vi "Dashboard Main.vi"() -> ()   [LabVIEW 2016]
uses:
  <vilib>/vision/Image Controls.llb/IMAQ Image.ctl
  Dashboard Tabs.ctl
  <vilib>/Utility/miscctls.llb/LVRowAndColumnTypeDef.ctl
  <vilib>/event_ctls.llb/eventvkey.ctl
  <vilib>/Rock Robotics/WPI/DriverStation/WPI_DriverStationRobotMode2.ctl
  <vilib>/Rock Robotics/Network Tables/NT Read Numeric Array.vi
  <vilib>/Rock Robotics/Network Tables/NT Read Boolean.vi
  <vilib>/Rock Robotics/Network Tables/NT Write Boolean.vi
  <vilib>/Rock Robotics/WPI/Dashboard/WPI_DashboardLogging Global.vi
  <vilib>/ptbypt/NI_PtbyPt.lvlib
  <vilib>/vision/NI_Vision_Development_Module.lvlib
panel:
  in  "output cluster":T2
  in  "Size Limit %":dbl=0.04
  in  "LED Color":T3={"Hue"={30.0, 150.0}, "Sat"={67.0, 194.28571428571428}, "Val"={49.0, 194.0}} {"Hue" scale=0.0..255.0 scale format="%#_3g"}
  in  "Camera 0 Brightness":dbl=5.0
  out "Camera Image 3":T1(plugin-control)
  out "Camera Image 2":T1(plugin-control)
  in  "Camera Settings Right":T4={"Frame Rate"=15, "Compression"=30, "Size"=2, "DB Camera Config"=FALSE} {"Frame Rate" scale=1.0..30.0; "Compression" scale=100.0..-1.0; "Size" items=["640x480", "320x240", "160x120"]}
  in  "Camera Name Right":string(combo)="Camera1"
  out "Camera Info":cluster{"Mbps LED":bool, "Mbps":dbl, "fps":dbl}={"Mbps LED"=FALSE, "Mbps"=0.1809963067335802, "fps"=11.600928074245939} {"fps" format="%#.1g"; "Mbps" format="%#.1g"}
  in  "Camera Settings":T4={"Frame Rate"=15, "Compression"=30, "Size"=2, "DB Camera Config"=FALSE} {"Frame Rate" scale=1.0..30.0; "Compression" scale=100.0..-1.0; "Size" items=["640x480", "320x240", "160x120"]}
  in  "TCP":refnum<k5>
  in  "Rec Mode":enum32{"Stop", "Record", "Playback"}(radio)
  out "Robot IP":string="10.10.38.2"
  out "Image Message":string="Timeout in Camera Communications"
  in  "Dashboard Tab":T5(tab)=enum."Cooler Stuff"
  in  "Select Auto":string(combo)="Select Autonomous ..."
  out "NT Connection":bool=TRUE
  out "MotorChart R":cluster{"Numeric":dbl, "Numeric":dbl}(graph)
  out "MotorChart L":cluster{"Numeric":dbl, "Numeric":dbl}(graph)
  out "MotorSliders R":cluster{"MotorSlide1":dbl, "MotorSlide2":dbl} {"MotorSlide2" scale=-1.0..1.0 scale format="%#_2e"; "MotorSlide1" scale=-1.0..1.0 scale format="%#_2e"}
  out "MotorSliders L":cluster{"MotorSlide1":dbl, "MotorSlide2":dbl} {"MotorSlide2" scale=-1.0..1.0 scale format="%#_2e"; "MotorSlide1" scale=-1.0..1.0 scale format="%#_2e"}
  out "Gyro":dbl(knob)=346.0 scale=0.0..360.0
  out "JS1 Z":dbl(slide) scale=-1.0..1.0 scale format="%#_2e"
  out "JS1 Graph":cluster{"X":dbl, "Y":dbl}[](graph)
  out "JS1 Buttons":T6
  out "JS2 Z":dbl(slide) scale=-1.0..1.0 scale format="%#_2e"
  out "JS2 Graph":cluster{"X":dbl, "Y":dbl}[](graph)=[{"X"=0.0, "Y"=-0.007874015748031496}]
  out "JS2 Buttons":T6
  out "Mode":T7(ring)
  in  "Recalibrate Gyro":bool
  in  "DB/String 9":string
  in  "DB/String 8":string
  in  "DB/String 7":string
  in  "DB/String 6":string
  in  "DB/String 5":string
  in  "DB/String 4":string
  in  "DB/String 3":string
  in  "DB/String 2":string
  in  "DB/String 1":string
  in  "DB/String 0":string
  in  "DB/Slider 0":dbl(slide) scale=0.0..5.0
  in  "DB/Slider 1":dbl(slide) scale=0.0..5.0
  in  "DB/Slider 2":dbl(slide) scale=0.0..5.0
  in  "DB/Slider 3":dbl(slide) scale=0.0..5.0
  out "DB/LED 3":bool
  out "DB/LED 2":bool
  out "DB/LED 1":bool
  out "DB/LED 0":bool
  in  "DB/Button 3":bool
  in  "DB/Button 2":bool
  in  "DB/Button 1":bool
  in  "DB/Button 0":bool caption="New Name"
  out "Results":T8 {"Score" format="%#_3g"; "Pixels"."Rectangle"."Numeric 5" format="%#_3g"; "Pixels"."Rectangle"."Numeric 3" format="%#_3g"; "Pixels"."Rectangle"."Numeric 2" format="%#_3g"; "Pixels"."Rectangle"."Numeric" format="%#_3g"; "Normalized"."Rectangle"."Numeric 5" format="%#_2g"; "Normalized"."Rectangle"."Numeric 3" format="%#_2g"; "Normalized"."Rectangle"."Numeric 2" format="%#_2g"; "Normalized"."Rectangle"."Numeric" format="%#_2g"; "Normalized"."Center"."?" format="%#_3g"; "Normalized"."Center"."?" format="%#_3g"; "Distance (ft)" format="%#_3g"}
  in  "Test Slider":dbl(slide) scale=0.0..100.0 scale format="%#_3g"
  in  "On/Off":bool caption="Solenoid"
  in  "Test Name":u16(ring) items=["Select the test to run..."]
  in  "Test Tree":string(tree)
  in  "Motor":cluster{"Value":dbl, "Enable":bool} {"Value" scale=-1.0..1.0 scale format="%#_3g"}
  out "Progress":T9 {"Test Progress" scale=0.0..100.0}
  in  "Rev/Fwd":cluster{"Forward":bool, "Reverse":bool}
  in  "Test Ring":u16(ring) items=["Monochrome", "Color"]
  out "Cmd Status":string
  in  "Execute Command":bool
  in  "Command Params":string[][](table)
  in  "Command Selection":i32(listbox)
  in  "CheckList":i32(listbox)
  out "Tree":string(tree)
  out "Ultrasonic (in.)":dbl
  in  "PID Shooter Baseline":dbl=0.62
  in  "Shooter Baseline":dbl=0.62
  in  "PID Shooter RPS":dbl=40.0
  out "Left Shooter Speed":dbl
  out "Gyro Value":dbl(knob)=346.0 scale=0.0..360.0
  out "Gear Door":bool
  out "PTO":bool
  out "Shooting Motor":bool
  out "Right Drive Speed":dbl
  out "Left Drive Speed":dbl
  out "Drive Mode":string="Dual Stick Arcade"
  out "Right Shooter Speed":dbl
  in  "Gyro Reset":bool
  out "Vision Particles":dbl
  out "Added Power":dbl=0.0007874015748031496 format="%#.2f"
  out "Shooter Mode":string="Raw Control"
  out "Right Motor:":dbl
  out "Conveyor":bool
  out "Shooting":bool
  out "Should this tab be open":bool
  out "Left Motor:":dbl
  out "Gyro Angle":dbl=346.0
  in  "Auton Select":T10(ring)
  out "Vision Particles: Auton":dbl
  out "Camera Image":T1(plugin-control)
  out "Background":bool
  in  "Camera Name":string(combo)="Camera0"
  # "HW"
  # "HW"
  # "Joysticks"
  # "Drive Motors"
  # "Front"
  # "Right"
  # "Left"
  # "Back"
  # "This tab is a great place for autonomous settings and robot-specific values.\nPlace controls and indicators inside this tab and match name to\nDashboard Variables on robot. You can also delete this comment."
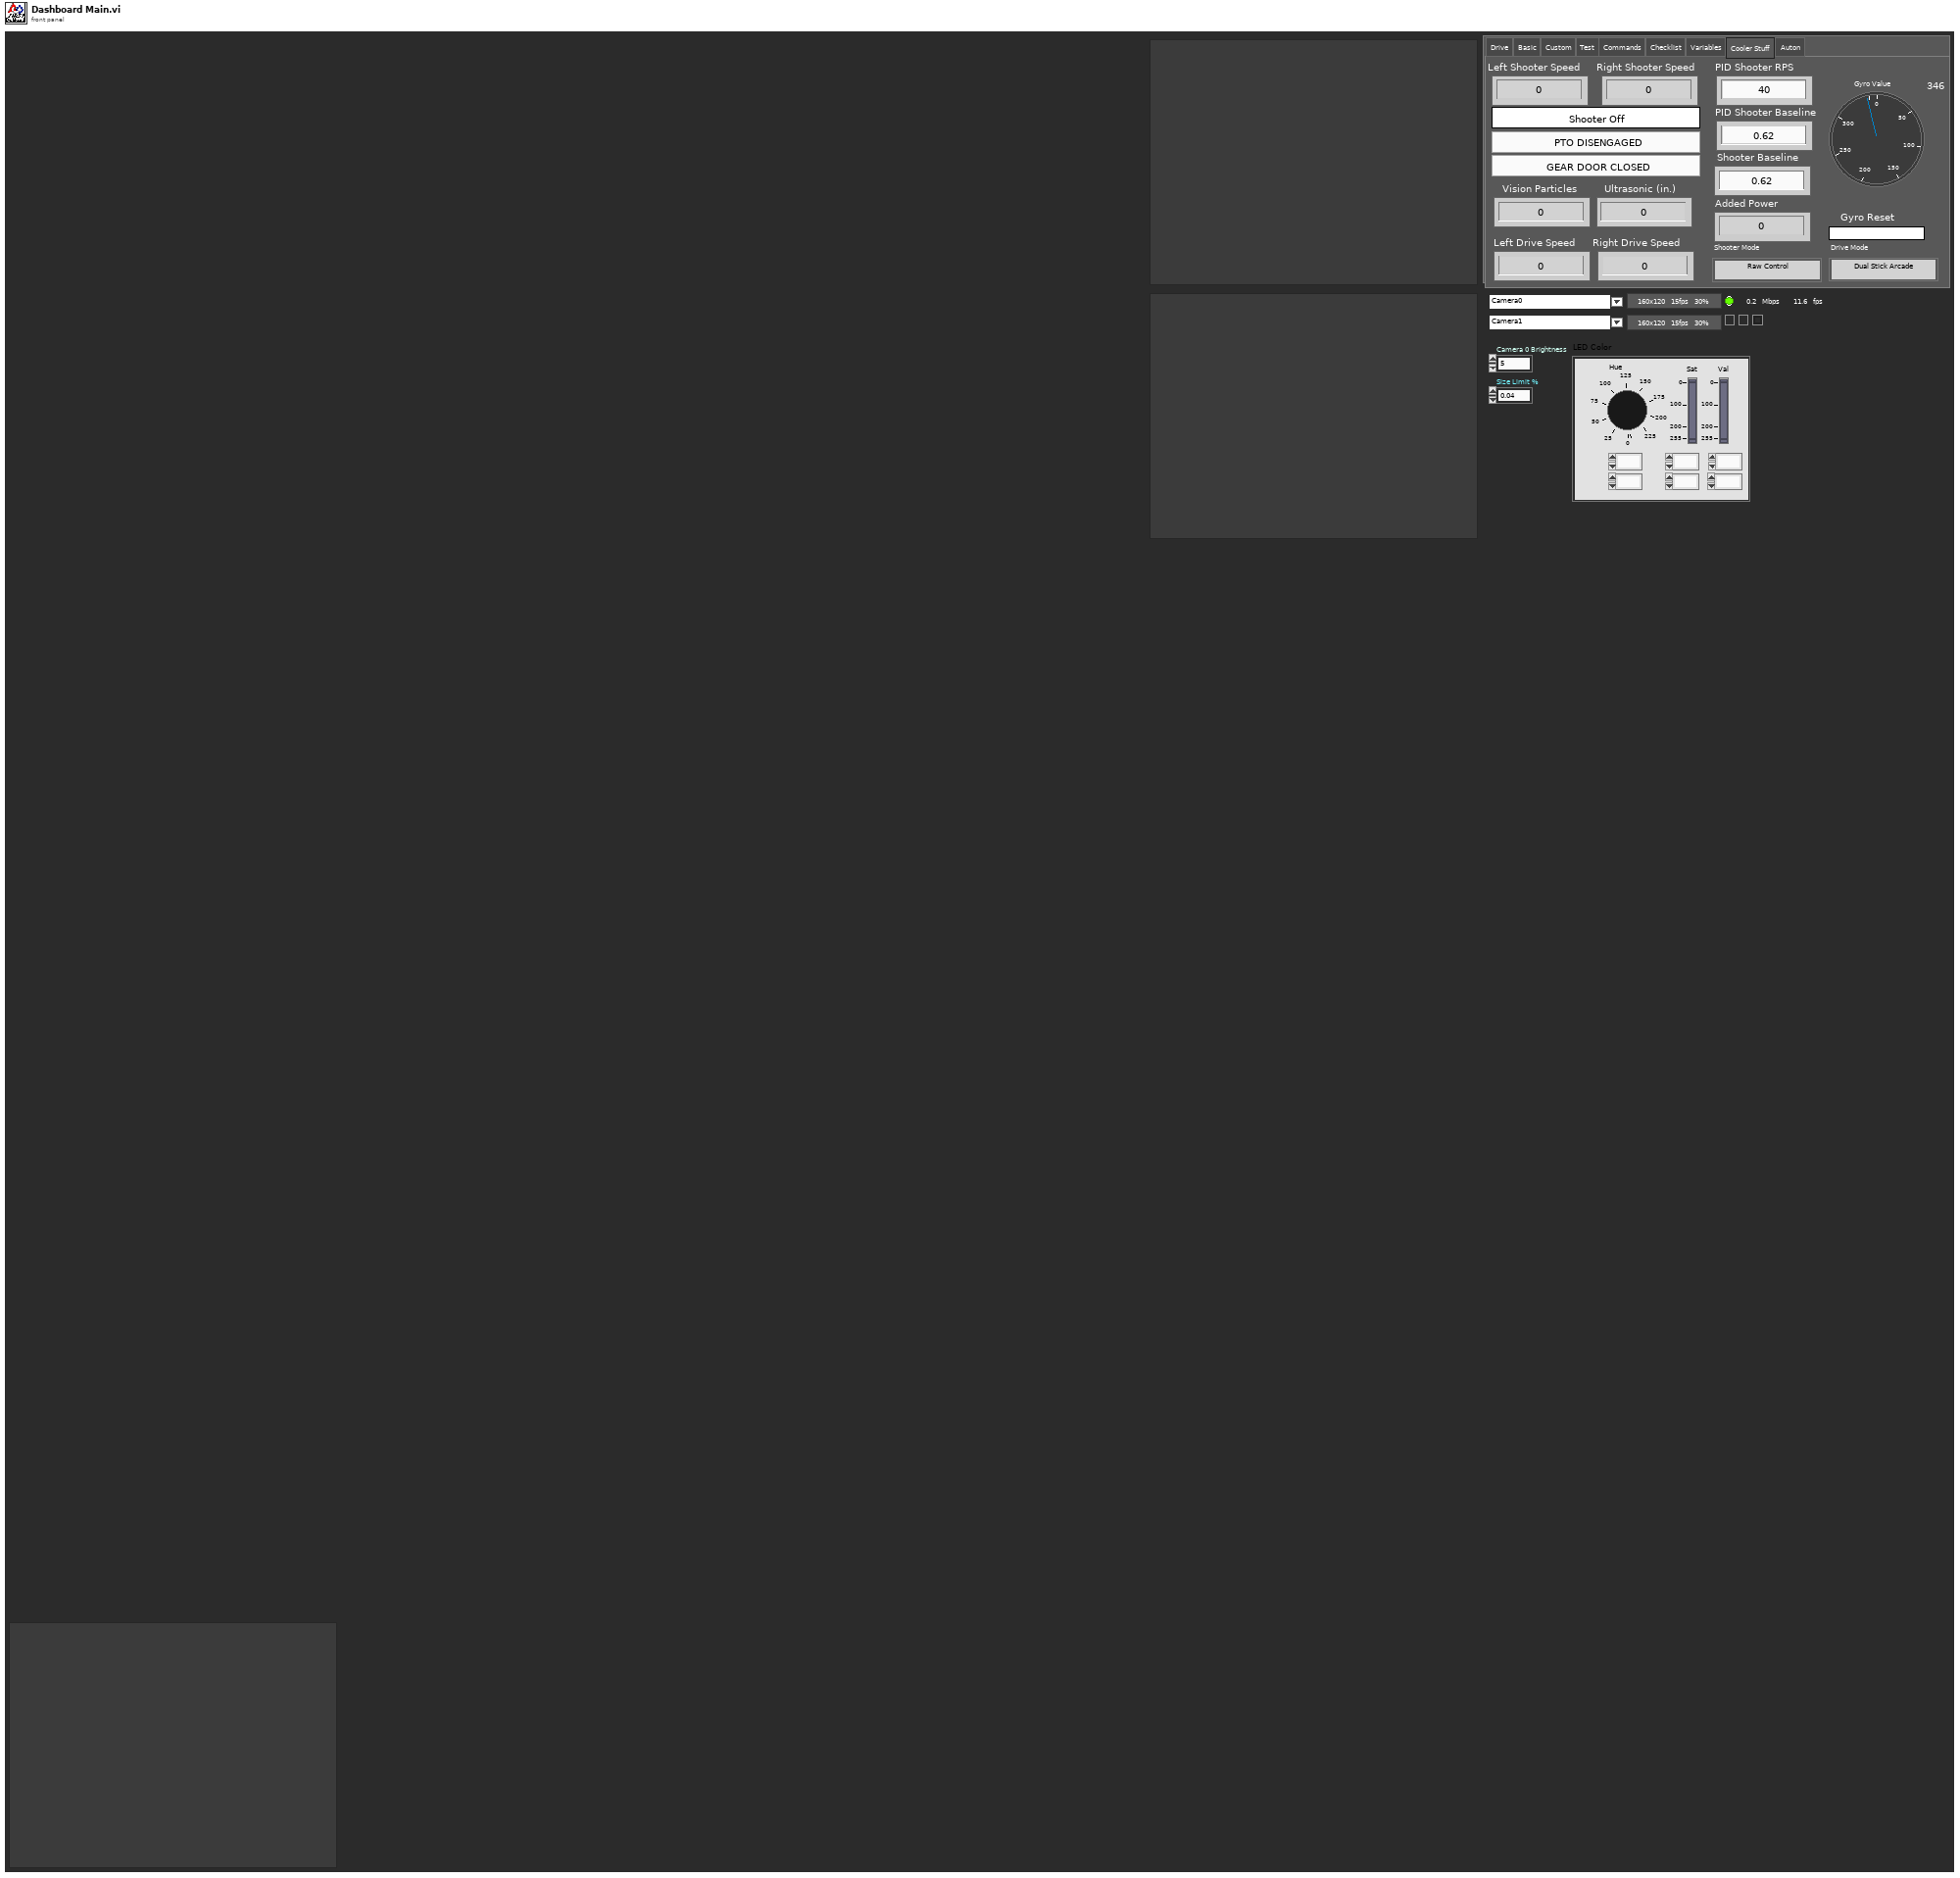
[diagram p1: front panel]
types:
  T1 = typedef "IMAQ Image.ctl" = refnum<image>
  T2 = cluster{"Image out":T1, "Results":cluster{"Distance (ft)":dbl, "Score":dbl, "Normalized":cluster{"Center":cluster{dbl, dbl}, "Rectangle":cluster{"Numeric":dbl, "Numeric 2":dbl, "Numeric 3":dbl, "Numeric 5":dbl}}, "Pixels":cluster{"Center":cluster{dbl, dbl}, "Rectangle":cluster{"Numeric":dbl, "Numeric 2":dbl, "Numeric 3":dbl, "Numeric 5":dbl}}}, "Edges":cluster{"X":sgl, "Y":sgl}[]}
  T3 = cluster{"Hue":cluster{dbl, dbl}, "Sat":cluster{dbl, dbl}, "Val":cluster{dbl, dbl}}
  T4 = cluster{"Frame Rate":i32, "Compression":i32, "Size":u16, "DB Camera Config":bool}
  T5 = enum32{"Drive", "Basic", "Custom", "Test", "Commands", "Checklist", "Variables", "Cooler Stuff", "Auton "}
  T6 = cluster{bool, bool, bool, bool, bool, bool, bool, bool, bool, bool, bool, bool}
  T7 = enum8{"Tele-Op Disabled", "Tele-Op Enabled", "Auto Disabled", "Auto Enabled", "Test Disabled", "Test Enabled", "Disconnected", "No Code", "E-Stop"}
  T8 = cluster{"Distance (ft)":dbl, "Score":dbl, "Normalized":cluster{"Center":cluster{dbl, dbl}, "Rectangle":cluster{"Numeric":dbl, "Numeric 2":dbl, "Numeric 3":dbl, "Numeric 5":dbl}}, "Pixels":cluster{"Center":cluster{dbl, dbl}, "Rectangle":cluster{"Numeric":dbl, "Numeric 2":dbl, "Numeric 3":dbl, "Numeric 5":dbl}}}
  T9 = cluster{"Test Progress":u8, "Test Progress Text":string}
  T10 = enum16{"Nothing", "Boiler Gear Auton", "Far Gear Auton", "Center Gear Auton", "Center Gear No Vision", "Center Gear Baseline Left", "Boiler Shoot", "Center Shoot", "Boiler Gear Shoot", "Center Gear Shoot", "Boiler Bucket Shoot", "Far Gear Bucket Cross", "Drive Straight"}
  T11 = typedef "Dashboard Tabs.ctl" = enum32{"Drive", "Basic", "Custom", "Test", "Commands", "Checklist", "Variables", "Cooler Stuff", "Auton "}
  T12 = typedef "Image Type" = u32
  T13 = cluster{"IDs":cluster{"RPC field ID":u16, "Unique ID":u16}, "String":string}
  T14 = enum32{"Drive", "Basic", "Custom", "Test", "Checklist", "Variables"}
  T15 = typedef "WPI_DriverStationRobotMode2.ctl" = enum16{"Autonomous Disabled", "Autonomous Enabled", "Teleop Disabled", "Teleop Enabled", "Disconnected", "Finish", "Test Disabled", "Test Enabled", "Emergency Stopped"}
  T16 = cluster{"Error Strings":string, "Disable Counts":cluster{u16, u16}, "Rail Faults":cluster{u16, u16, u16}, "Robot IP":string, "DB Mode":u8, "Event Info":cluster{"Name":string, "Type":u8, "Number":u16, "Replay":u8}}
  T17 = cluster{"Storage":cluster{"Disk Free":u64, "RAM Block":u32, "RAM free":u32}, "CPU Utilization":cluster{"CPU % ISR":sgl, "CPU % Time Crit":sgl, "CPU % Timed Str":sgl, "CPU % High":sgl, "CPU % Above":sgl, "CPU % Normal":sgl, "CPU % Low":sgl}, "CAN":cluster{"% Bus Utilization":sgl, "Bus Off Cnt":u32, "TX_FIFO Full Cnt":u32, "Receive Error Cnt":u8, "Transmit Error Cnt":u8}, "HID":cluster{"HID Outputs":u32, "Rumble Low":u16, "Rumble High":u16}[]}
  T18 = cluster{"Status bits":cluster{"Test Mode":bool, "Autonomous":bool, "Enabled":bool, "Code Start":bool, "Brownout":bool, "Reserved 2":bool, "Reserved 3":bool, "E-Stop":bool}, "Code Trace":cluster{"Disabled":bool, "TeleOp":bool, "Auto":bool, "Test":bool}, "Controller Type":enum16{"unknown", "cRIO", "roboRio"}, "Code?":enum16{"unknown", "noCode", "code"}, "Battery V":dbl}
  T19 = cluster{"Control Bits":cluster{"TestMode":bool, "Autonomous":bool, "Enabled":bool, "FMS Present":bool, bool, bool, bool, "E-Stop":bool}, "Team Station ":u8, "Countdown":sgl, "Joystick Values":cluster{"Axes":dbl[], "Buttons":bool[], "POVs":i16[]}[]}
  T20 = cluster{"Axes":dbl[], "Buttons":bool[], "POVs":i16[]}[]
  T21 = cluster{"Axes":dbl[], "Buttons":bool[], "POVs":i16[]}
  T22 = cluster{"Buttons[0]":bool, "Buttons[1]":bool, "Buttons[2]":bool, "Buttons[3]":bool, "Buttons[4]":bool, "Buttons[5]":bool, "Buttons[6]":bool, "Buttons[7]":bool, "Buttons[8]":bool, "Buttons[9]":bool, "Buttons[10]":bool, "Buttons[11]":bool}
  T23 = cluster{"Camera Image":refnum<vi>, "Dashboard Tab":refnum<vi>, "Background":refnum<vi>, "Rec Mode":refnum<vi>, "Test Slider":refnum<vi>, "On/Off ":refnum<vi>, "Test Ring":refnum<vi>, "Rev/Fwd":refnum<vi>, "Test Name":refnum<vi>, "Motor":refnum<vi>, "Progress":refnum<vi>, "CheckList":refnum<vi>, "Tree":refnum<vi>, "Test Tree":refnum<vi>, "Command Params":refnum<vi>, "Command Selection":refnum<vi>, "Execute Command":refnum<vi>, "Cmd Status":refnum<vi>, "Camera Settings":refnum<vi>, "Camera Name":refnum<vi>, "Camera Info":refnum<vi>, "Camera Settings Right":refnum<vi>, "Camera Name Right":refnum<vi>, "Camera Image":refnum<vi>}
  T24 = cluster{"Operation":enum16{"Update", "Clear"}, "Color Box":u32}[]
  T25 = typedef "eventvkey.ctl" = enum16{"ASCII", "Enter", "Return", "Shift", "Ctrl", "Alt", "Cmd", "Opt", "Caps", "NumLock", "Clear", "Break", "Up", "Down", "Left", "Right", "Insert", "Delete", "Home", "End", "PageUp", "PageDown", "Escape", "Help", "Pause", "ScrollLock", "F1", "F2", "F3", "F4", "F5", "F6", "F7", "F8", "F9", "F10", "F11", "F12", "F13", "F14", "F15", "F16", "F17", "F18", "F19", "F20", "F21", "F22", "F23", "F24", "Play", "VolumeUp", "VolumeDown", "Mute", "Two Byte Char"}
  T26 = cluster{"Image Size":bool, "Image Type":bool, "Pixel Value":bool, "ROI Information":bool, "Zoom Factor":bool}
  T27 = cluster{"Operation":enum16{"Update", "Clear"}, "Color Box":u32}
  T28 = typedef "LVRowAndColumnTypeDef.ctl" = cluster{"Row":i32, "Column":i32}
  T29 = cluster{"Shift":bool, "Ctrl":bool, "Alt":bool, "Cmd":bool, "Opt":bool}
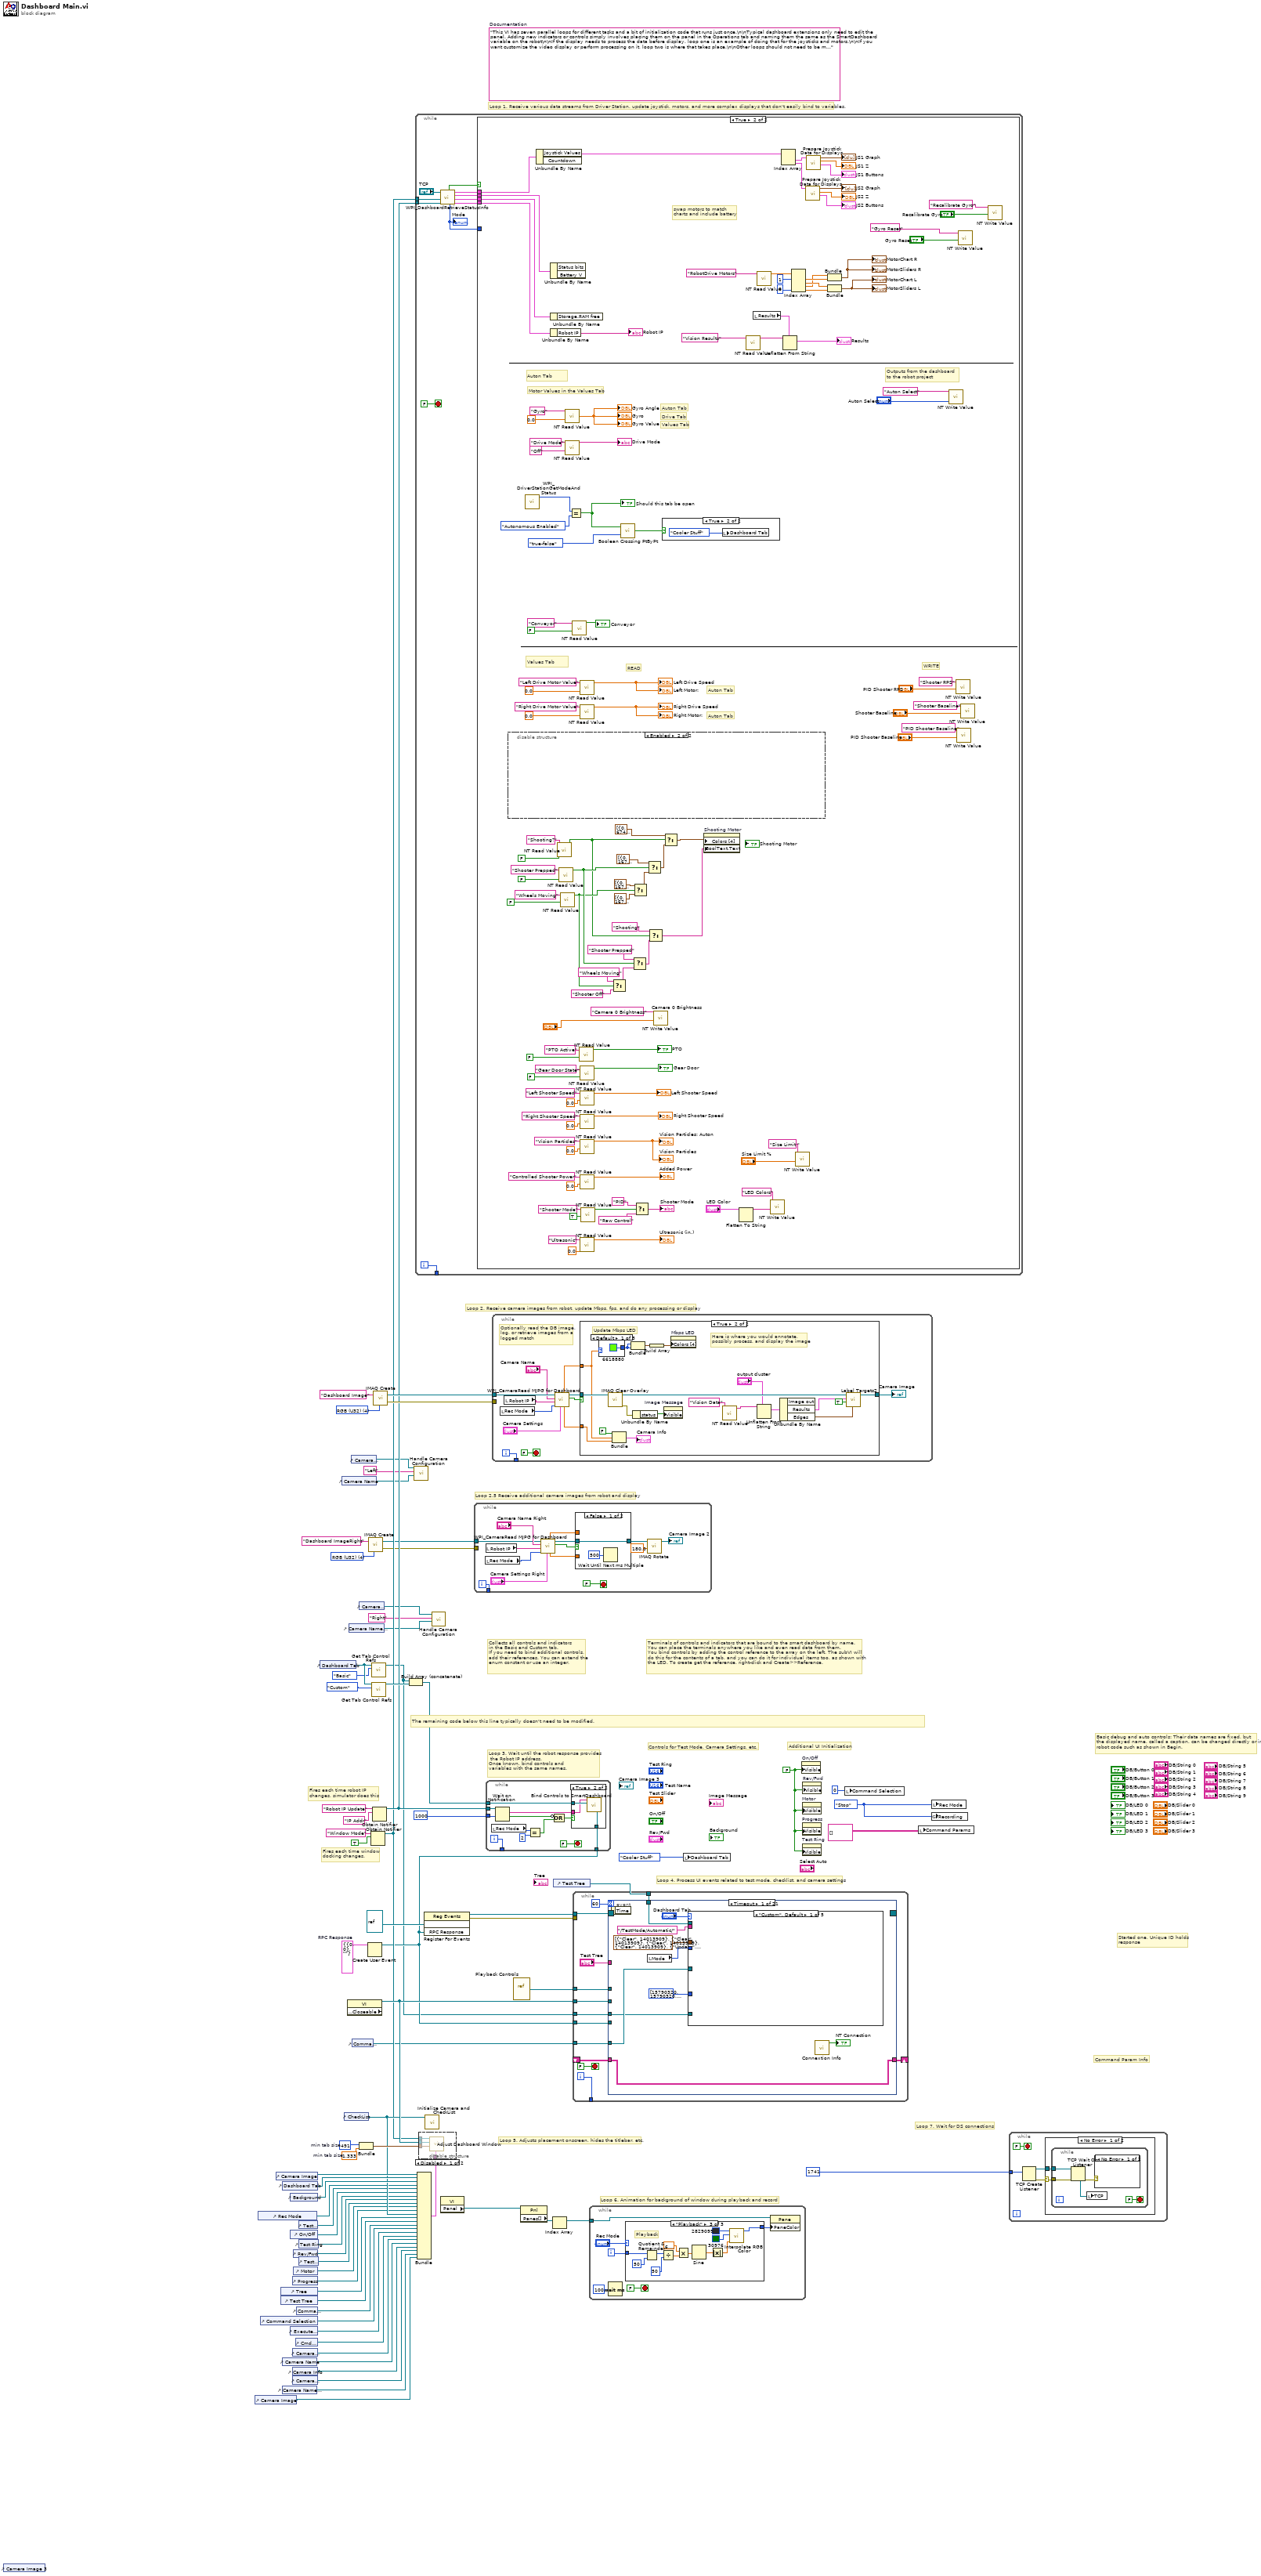
[diagram p0: block diagram]
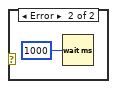
[diagram p4: hidden frame]
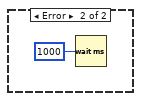
[diagram p5: hidden frame]
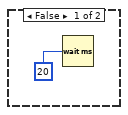
[diagram p6: hidden frame]
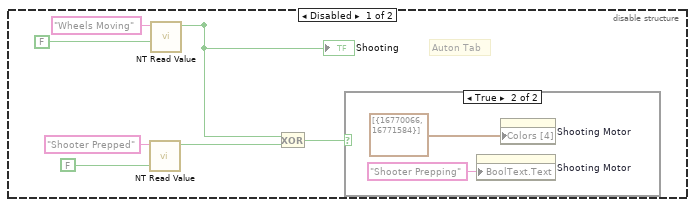
[diagram p7: hidden frame]
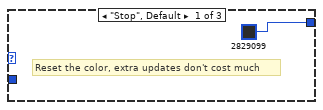
[diagram p10: hidden frame]
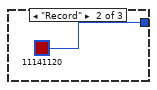
[diagram p11: hidden frame]
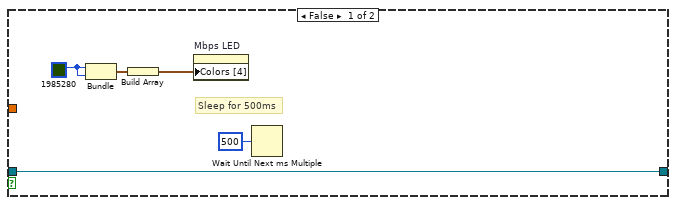
[diagram p13: hidden frame]
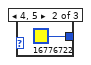
[diagram p14: hidden frame]
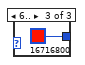
[diagram p15: hidden frame]
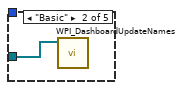
[diagram p16: hidden frame]
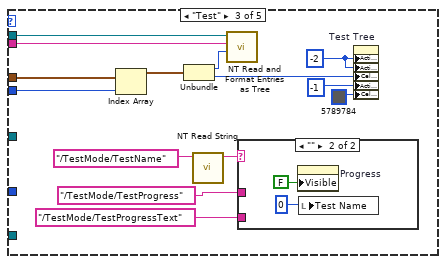
[diagram p17: hidden frame]
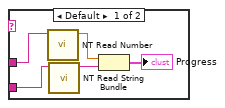
[diagram p18: hidden frame]
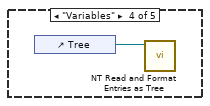
[diagram p19: hidden frame]
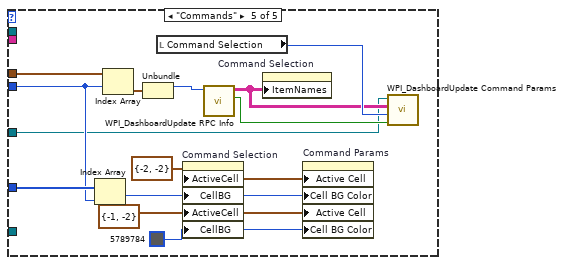
[diagram p20: hidden frame]
diagram:
  w11 = T12 4 items=["Grayscale (U8)", "Grayscale (I16)", "Grayscale (SGL)", "Complex (CSG)", "RGB (U32)", "HSL (U32)", "RGB (U64)"] ("Image Type")
  w25 = T13 {"IDs"={"RPC field ID"=0, "Unique ID"=0}, "String"=""}  # RPC Response
  w49 = 491  # min tab size
  w48 = 1.333  # min tab size
  w56 = enum32{"Stop", "Record", "Playback"}."Stop" ("Rec Mode")
  w31 = FALSE ("Visible")
  (unwired) "This VI has seven parallel loops for different tasks and a bit of initialization code that runs just once.\n\nTypical dashboard extensions only need to edit the panel. Adding new indicators or controls simply involves placing them on the panel in the Operations tab and naming them the same as the SmartDashboard variable on the robot\n\nIf the display needs to process the data before display, loop one is an example of doing that for the joysticks and motors.\n\nIf you want customize the video display or perform processing on it, loop two is where that takes place.\n\nOther loops should not need to be modified. They are pretty standard, and document the task they perform."  # Documentation
  w73 = T12 4 items=["Grayscale (U8)", "Grayscale (I16)", "Grayscale (SGL)", "Complex (CSG)", "RGB (U32)", "HSL (U32)", "RGB (U64)"] ("Image Type")
  # "Loop 2.5 Receive additional camera images from robot and display"
  # "Command Param Info"
  # "Started one, Unique ID holds\nresponse"
  # "Loop 7. Wait for DS connections"
  # "Basic debug and auto controls: Their data names are fixed, but\nthe displayed name, called a caption, can be changed directly or in\nrobot code such as shown in Begin."
  # "Controls for Test Mode, Camera Settings, etc."
  # "Additional UI Initialization"
  # "Loop 6. Animation for background of window during playback and record"
  # "Fires each time robot IP\nchanges, simulator does this"
  # "Fires each time window\ndocking changes."
  # "Collects all controls and indicators\nin the Basic and Custom tab.\nIf you need to bind additional controls,\nadd their references. You can extend the\nenum constant or use an integer."
  # "The remaining code below this line typically doesn't need to be modified."
  # "Loop 4. Process UI events related to test mode, checklist, and camera settings"
  # "Terminals of controls and indicators that are bound to the smart dashboard by name.\nYou can place the terminals anywhere you like and even read data from them.\nYou bind controls by adding the control reference to the array on the left. The subVI will\ndo this for the contents of a tab, and you can do it for individual items too, as shown with\nthe LED. To create get the reference, right-click and Create>>Reference."
  # "Loop 3. Wait until the robot response provides\n the Robot IP address.\nOnce known, bind controls and\nvariables with the same names."
  # "Loop 5. Adjusts placement onscreen, hides the titlebar, etc."
  # "Loop 1. Receive various data streams from Driver Station, update joystick, motors, and more complex displays that don't easily bind to variables."
  # "Loop 2. Receive camera images from robot, update Mbps, fps, and do any processing or display"
  n1 = control-ref of="Camera Image 3"() -> ()  [unwired: 1 out]
  n2 = control-ref of="Camera Image"() -> (w2:refnum<vi>)
  n3 = control-ref of="Rec Mode"() -> (w37:refnum<vi>)
  n4 = control-ref of="Command Selection"() -> (w24:refnum<vi>)
  n5 = control-ref of="Camera Image"() -> (w51:refnum<vi>)
  n6 = control-ref of="Tree"() -> (w41:refnum<vi>)
  n7 = control-ref of="Test Tree"() -> (w40:refnum<vi>)
  n8 = control-ref of="Dashboard Tab"() -> (w50:refnum<vi>)
  n9 = control-ref of="Camera Name"() -> (w15:refnum<vi>)
  n10 = control-ref of="Camera Name Right"() -> (w3:refnum<vi>)
  n11 = control-ref of="Execute Command"() -> (w26:refnum<vi>)
  n12 = control-ref of="Background"() -> (w46:refnum<vi>)
  n13 = control-ref of="On/Off"() -> (w35:refnum<vi>)
  n14 = control-ref of="Progress"() -> (w32:refnum<vi>)
  n15 = control-ref of="Camera Settings"() -> (w16:refnum<vi>)
  n16 = control-ref of="Camera Info"() -> (w14:refnum<vi>)
  n17 = control-ref of="Camera Settings Right"() -> (w4:refnum<vi>)
  n18 = control-ref of="Rev/Fwd"() -> (w33:refnum<vi>)
  n19 = control-ref of="Motor"() -> (w38:refnum<vi>)
  n20 = control-ref of="Cmd Status"() -> (w20:refnum<vi>)
  n21 = control-ref of="Command Params"() -> (w27:refnum<vi>)
  n22 = control-ref of="Test Slider"() -> (w36:refnum<vi>)
  n23 = control-ref of="Test Ring"() -> (w34:refnum<vi>)
  n24 = control-ref of="Test Name"() -> (w39:refnum<vi>)
  n25 = control-ref of="Dashboard Tab"() -> (w54:refnum<vi>)
  n26 = control-ref of="Camera Name"() -> (w17:refnum<vi>)
  n27 = control-ref of="CheckList"() -> (w42:refnum<vi>)
  n28 = property class="VI" props=["Front Panel.Closeable"]() -> (reference out=w55:refnum<vi>)  [unwired: 2 in, 2 out]
  n29 = control-ref of="Camera Name Right"() -> (w7:refnum<vi>)
  n30 = control-ref of="Camera Settings"() -> (w18:refnum<vi>)
  n31 = control-ref of="Command Params"() -> (w19:refnum<vi>)
  n32 = control-ref of="Camera Settings Right"() -> (w8:refnum<vi>)
  n33 = Bundle("min tab size"=w49, "min tab size"=w48) -> (w47:cluster{"min tab size":i32, "min tab size":dbl})  [unwired: 1 in]
  n34 = Create User Event(user event datatype=w25) -> (user event=w21:refnum<user-event>)  [unwired: 1 in, 1 out]
  n35 = call "IMAQ Create"("Image Name"="Dashboard ImageRight", "Image Type"=w11) -> ("New Image"=w10:T1, "error out"=w9:errorcluster)  [unwired: 2 in, 1 out]
  n36 = Obtain Notifier(name (unnamed)="Window Mode", notification data type=TRUE) -> (notifier out=w29:refnum<notifier>)  [unwired: 2 in, 2 out]
  n37 = call <vilib>:"Get Tab Control Refs.vi"("Page Index"=T14."Basic" ("Dashboard Tab"), "TabControl in"=w54) -> ("ControlsOnPage"=w13:refnum<vi>[])  [unwired: 9 in]
  n38 = call <vilib>:"Get Tab Control Refs.vi"("Page Index"=T14."Custom" ("Dashboard Tab"), "TabControl in"=w54) -> ("ControlsOnPage"=w53:refnum<vi>[])  [unwired: 9 in]
  n39 = Obtain Notifier(name (unnamed)="Robot IP Update", notification data type="IP Addr" ("name (unnamed)")) -> (notifier out=w30:refnum<notifier>)  [unwired: 2 in, 2 out]
  n40 = call "IMAQ Create"("Image Name"="Dashboard Image", "Image Type"=w73) -> ("New Image"=w71:T1, "error out"=w70:errorcluster)  [unwired: 2 in, 1 out]
  n41 = Build Array (concatenate)(w13, w53) -> (w52:refnum<vi>[])
  n42 = call "Handle Camera Configuration.vi"("CameraNameRef"=w17, "Camera File Name"="Left", "ClusterRef"=w18) -> ()  [unwired: 9 in]
  n43 = while {
    tunnel: [w83] -> _
    tunnel: w30 -> [w77]
    tunnel: w29 -> [w74]
    i -> [w83]
    stop <- FALSE stop-if-true
    n44 = call <vilib>:"WPI_DashboardRetrieveStatusInfo.vi"("Binding Refnum"=w77, "Window Mode Notifier"=w74, "TCP Cnx"="TCP") -> ("Power and Errors"=w78:T16, "Robot Metrics"=w81:T17, "Status Info"=w82:T18, "Control Info"=w79:T19, "Robot Mode"=w76:T7, "Process?"=w80:bool)  [unwired: 3 in]
    "Mode" <- w76
    n45 = case shown="True" w80 {
      tunnel: w82 -> [_ w202]
      tunnel: w81 -> [_ w201]
      tunnel: w79 -> [_ w200]
      tunnel: w78 -> [_ w199]
      tunnel: w76 -> [_ _]
      frame False {
        n46 = Wait (ms)(milliseconds to wait=u32 20) -> ()  [unwired: 1 out]
      }
      frame True {
        # "WRITE"
        # "READ"
        # "Outputs from the dashboard \nto the robot project"
        # "Motor Values in the Values Tab"
        # "Auton Tab"
        # "Auton Tab"
        # "Values Tab"
        # "Auton Tab"
        # "Drive Tab"
        # "Values Tab"
        # "Auton Tab"
        # "swap motors to match\ncharts and include battery"
        n47 = disable-structure shown="Enabled" {
          frame Disabled {
            # "Auton Tab"
            n48 = call-poly <vilib>:"NT Read Value.vi"("Default Value"=FALSE, "Name"="Shooter Prepped") -> ("Boolean"=w204:bool)  [unwired: 8 in, 1 out]
            n49 = call-poly <vilib>:"NT Read Value.vi"("Default Value"=FALSE, "Name"="Wheels Moving") -> ("Boolean"=w205:bool)  [unwired: 8 in, 1 out]
            "Shooting" <- w205
            n50 = Exclusive Or(1:w204, 2:w205) -> (0:w203:bool)
            n51 = case shown="True" w203 {
              frame False {
              }
              frame True {
                n52 = property on="Shooting Motor" class="Bool (strict)"("BoolText.Text"="Shooter Prepping" ("Boolean Text.Text")) -> ()  [unwired: 2 in, 2 out]
                n53 = property on="Shooting Motor" class="Bool (strict)"("Colors [4]"=cluster{u32, u32}[] [{16770066, 16771584}]) -> ()  [unwired: 2 in, 2 out]
              }
            }
          }
          frame Enabled {
          }
        }
        n54 = call <vilib>:"WPI_DriverStationGetModeAndStatus.vi"() -> ("Robot Mode"=w119:T15)  [unwired: 10 in, 1 out]
        n55 = Unbundle By Name(w200) -> ("Joystick Values"=w190:T20)  [unwired: 1 out]
        n56 = Unbundle By Name(w202) -> ()  [unwired: 2 out]
        n57 = Unbundle By Name(w201) -> ()  [unwired: 1 out]
        n58 = Unbundle By Name(w199) -> ("Robot IP"=→"Robot IP":string)
        n59 = call-poly <vilib>:"NT Read Value.vi"("Default Value"=FALSE, "Name"="Shooting?") -> ("Boolean"=w126:bool)  [unwired: 8 in, 1 out]
        n60 = call-poly <vilib>:"NT Read Value.vi"("Default Value"=FALSE, "Name"="Shooter Prepped") -> ("Boolean"=w128:bool)  [unwired: 8 in, 1 out]
        n61 = call-poly <vilib>:"NT Read Value.vi"("Default Value"=FALSE, "Name"="Wheels Moving") -> ("Boolean"=w127:bool)  [unwired: 8 in, 1 out]
        n62 = call-poly <vilib>:"NT Read Value.vi"("Default Value"=0.0, "Name"="Gyro") -> ("Numeric"=→"Gyro" →"Gyro Angle" →"Gyro Value":dbl)  [unwired: 8 in, 1 out]
        n63 = call-poly <vilib>:"NT Read Value.vi"("Default Value"="Off", "Name"="Drive Mode") -> ("String"=→"Drive Mode":string)  [unwired: 8 in, 1 out]
        n64 = Equal?(x=w119, y=WPI_DriverStationRobotMode2."Autonomous Enabled" ("Robot Mode")) -> (x = y?=w118:bool)
        "Should this tab be open" <- w118
        n65 = call-poly <vilib>:"NT Read Value.vi"("Default Value"=FALSE, "Name"="Conveyor") -> ("Boolean"=→"Conveyor":bool)  [unwired: 8 in, 1 out]
        n66 = call-poly <vilib>:"NT Read Value.vi"("Default Value"=FALSE, "Name"="PTO Active") -> ("Boolean"=→"PTO":bool)  [unwired: 8 in, 1 out]
        n67 = call-poly <vilib>:"NT Read Value.vi"("Default Value"=0.0, "Name"="Left Drive Motor Value") -> ("Numeric"=→"Left Motor:" →"Left Drive Speed":dbl)  [unwired: 8 in, 1 out]
        n68 = call-poly <vilib>:"NT Read Value.vi"("Default Value"=0.0, "Name"="Right Drive Motor Value") -> ("Numeric"=→"Right Drive Speed" →"Right Motor:":dbl)  [unwired: 8 in, 1 out]
        n69 = call-poly <vilib>:"NT Read Value.vi"("Default Value"=FALSE, "Name"="Gear Door State") -> ("Boolean"=→"Gear Door":bool)  [unwired: 8 in, 1 out]
        n70 = call-poly <vilib>:"NT Read Value.vi"("Default Value"=0.0, "Name"="Left Shooter Speed") -> ("Numeric"=→"Left Shooter Speed":dbl)  [unwired: 8 in, 1 out]
        n71 = call-poly <vilib>:"NT Read Value.vi"("Default Value"=0.0, "Name"="Right Shooter Speed") -> ("Numeric"=→"Right Shooter Speed":dbl)  [unwired: 8 in, 1 out]
        n72 = call-poly <vilib>:"NT Read Value.vi"("Default Value"=0.0, "Name"="Vision Particles") -> ("Numeric"=→"Vision Particles: Auton" →"Vision Particles":dbl)  [unwired: 8 in, 1 out]
        n73 = call-poly <vilib>:"NT Read Value.vi"("Default Value"=0.0, "Name"="Controlled Shooter Power") -> ("Numeric"=→"Added Power":dbl)  [unwired: 8 in, 1 out]
        n74 = call-poly <vilib>:"NT Read Value.vi"("Default Value"=0.0, "Name"="Ultrasonic") -> ("Numeric"=→"Ultrasonic (in.)":dbl)  [unwired: 8 in, 1 out]
        n75 = call-poly <vilib>:"NT Read Value.vi"("Default Value"=TRUE, "Name"="Shooter Mode") -> ("Boolean"=w99:bool)  [unwired: 8 in, 1 out]
        n76 = Select(t="Wheels Moving", s=w127, f="Shooter Off") -> (s? t:f=w130:string)
        n77 = call <vilib>:"Boolean Crossing PtByPt.vi"("direction"=enum16{"either", "false-true", "true-false"}."true-false", "input"=w118) -> ("crossing"=w167:bool)  [unwired: 1 in]
        n78 = Select(t="Shooter Prepped", s=w128, f=w130) -> (s? t:f=w129:string)
        n79 = Select(t=cluster{u32, u32}[] [{0, 16728642}] ("Colors [4]"), s=w127, f=cluster{u32, u32}[] [{0, 16777215}] ("Colors [4]")) -> (s? t:f=w137:cluster{u32, u32}[])
        n80 = Select(t="PID", s=w99, f="Raw Control") -> (s? t:f=→"Shooter Mode":string)
        n81 = Select(t=cluster{u32, u32}[] [{0, 16776722}] ("Colors [4]"), s=w128, f=w137) -> (s? t:f=w136:cluster{u32, u32}[])
        n82 = Select(t="Shooting", s=w126, f=w129) -> (s? t:f=w125:string)
        n83 = call-poly <vilib>:"NT Write Value.vi"("Numeric"="Camera 0 Brightness", "Name"="Camera 0 Brightness") -> ()  [unwired: 9 in, 1 out]
        n84 = case shown="True" w167 {
          frame False {
          }
          frame True {
            n85 = local write "Dashboard Tab"(Dashboard_Tabs."Cooler Stuff" ("Dashboard Tab")) -> ()
          }
        }
        n86 = Select(t=cluster{u32, u32}[] [{0, 6749952}] ("Colors [4]"), s=w126, f=w136) -> (s? t:f=w131:cluster{u32, u32}[])
        n87 = property on="Shooting Motor" class="Bool (strict)"("Colors [4]"=w131, "BoolText.Text"=w125) -> ()  [unwired: 2 in, 2 out]
        n88 = Flatten To String(anything="LED Color") -> (data string=w91:string)  [unwired: 3 in, 2 out]
        n89 = call-poly <vilib>:"NT Read Value.vi"("Name"="Vision Results") -> ("String"=w172:string)  [unwired: 9 in, 1 out]
        n90 = local read "Results"() -> (w171:T8)
        n91 = call-poly <vilib>:"NT Read Value.vi"("Name"="RobotDrive Motors") -> ("Numeric Array"=w180:dbl[])  [unwired: 9 in, 1 out]
        n92 = call-poly <vilib>:"NT Write Value.vi"("String"=w91, "Name"="LED Colors") -> ()  [unwired: 9 in, 1 out]
        n93 = Index Array(array=w190) -> (element #1=w189:T21, element #2=w185:T21)  [unwired: 2 in]
        n94 = Unflatten From String(type=w171, binary string=w172) -> (value=→"Results":T8)  [unwired: 3 in, 2 out]
        n95 = Index Array(array=w180, index #1=1, index #4=0) -> (element #1=w194:dbl, element #2=w195:dbl, element #3=w193:dbl, element #4=w198:dbl)  [unwired: 2 in]
        n96 = call-poly <vilib>:"NT Write Value.vi"("Numeric"="Size Limit %", "Name"="Size Limit ") -> ()  [unwired: 9 in, 1 out]
        n97 = call "Prepare Joystick Data for Displays.vi"("Joystick Values"=w185) -> ("Buttons"=→"JS2 Buttons":T22, "Z Axis"=→"JS2 Z":dbl, "Cartesian Data"=→"JS2 Graph":cluster{"X axis":dbl, "X axis":dbl}[])  [unwired: 8 in]
        n98 = call "Prepare Joystick Data for Displays.vi"("Joystick Values"=w189) -> ("Buttons"=→"JS1 Buttons":T22, "Z Axis"=→"JS1 Z":dbl, "Cartesian Data"=→"JS1 Graph":cluster{"X axis":dbl, "X axis":dbl}[])  [unwired: 8 in]
        n99 = Bundle("Numeric"=w193, "Numeric"=w194) -> (→"MotorChart R" →"MotorSliders R":cluster{"Numeric":dbl, "Numeric":dbl})  [unwired: 1 in]
        n100 = Bundle("Numeric"=w195, "Numeric"=w198) -> (→"MotorChart L" →"MotorSliders L":cluster{"Numeric":dbl, "Numeric":dbl})  [unwired: 1 in]
        n101 = call-poly <vilib>:"NT Write Value.vi"("Numeric"="Auton Select", "Name"="Auton Select") -> ()  [unwired: 9 in, 1 out]
        n102 = call-poly <vilib>:"NT Write Value.vi"("Numeric"="PID Shooter RPS", "Name"="Shooter RPS") -> ()  [unwired: 9 in, 1 out]
        n103 = call-poly <vilib>:"NT Write Value.vi"("Numeric"="PID Shooter Baseline", "Name"="PID Shooter Baseline") -> ()  [unwired: 9 in, 1 out]
        n104 = call-poly <vilib>:"NT Write Value.vi"("Boolean"="Gyro Reset", "Name"="Gyro Reset") -> ()  [unwired: 9 in, 1 out]
        n105 = call-poly <vilib>:"NT Write Value.vi"("Numeric"="Shooter Baseline", "Name"="Shooter Baseline") -> ()  [unwired: 9 in, 1 out]
        n106 = call-poly <vilib>:"NT Write Value.vi"("Boolean"="Recalibrate Gyro", "Name"="Recalibrate Gyro") -> ()  [unwired: 9 in, 1 out]
      }
    }
  }
  n107 = Bundle("Camera Image"=w51, "Dashboard Tab"=w50, "Background"=w46, "Rec Mode"=w37, "Test Slider"=w36, "On/Off"=w35, "Test Ring"=w34, "Rev/Fwd"=w33, "Test Name"=w39, "Motor"=w38, "Progress"=w32, "CheckList"=w42, "Tree"=w41, "Test Tree"=w40, "Command Params"=w27, "Command Selection"=w24, "Execute Command"=w26, "Cmd Status"=w20, "Camera Settings"=w16, "Camera Name"=w15, "Camera Info"=w14, "Camera Settings Right"=w4, "Camera Name Right"=w3, "Camera Image"=w2) -> (w43:T23)  [unwired: 1 in]
  n108 = disable-structure shown="Disabled" {
    disable-tunnel: w55 -> [w216 _]
    disable-tunnel: w47 -> [w215 _]
    disable-tunnel: w43 -> [w214 _]
    disable-tunnel: w29 -> [w213 _]
    frame Disabled {
      n109 = call "Adjust Dashboard Window.vi"("Sizing Refnums"=w214, "Size Constraints"=w215, "VI"=w216, "WIn Mode"=w213) -> ()  [unwired: 8 in]
    }
    frame Enabled {
    }
  }
  n110 = register-events(refnum<vi> refnum, w21) -> (reference out=w60:refnum<event-registration>, error out=w59:errorcluster)  [unwired: 2 in]
  n111 = call "Initialize Camera and CheckList.vi"("ListBox in"=w42) -> ()  [unwired: 11 in]
  n112 = call "Handle Camera Configuration.vi"("CameraNameRef"=w7, "Camera File Name"="Right", "ClusterRef"=w8) -> ()  [unwired: 9 in]
  n113 = property class="VI"() -> ("Panel"=w63:refnum<vi>)  [unwired: 2 in, 2 out]
  n114 = while {
    tunnel: w10 -> [w229]
    tunnel: w9 -> [_]
    tunnel: [w223] -> _
    i -> [w223]
    stop <- FALSE stop-if-true
    n115 = local read "Rec Mode"() -> (w227:enum32{"Stop", "Record", "Playback"})
    n116 = local read "Robot IP"() -> (w228:string)
    n117 = call <vilib>:"WPI_CameraRead MJPG for Dashboard.vi"("Camera Settings"="Camera Settings Right", "Rec Mode"=w227, "Robot IP"=w228, "Camera Name"="Camera Name Right", "Refnum in"=w229) -> ("Active"=w222:bool, "Refnum out"=w225:T1, "FPS"=w220:dbl, "Bandwidth (Mbps)"=w221:dbl)  [unwired: 3 in]
    n118 = case shown="False" w222 {
      tunnel: w225 -> [w231 w233]
      tunnel: w221 -> [_ _]
      tunnel: w220 -> [_ _]
      tunnel: [w231 w233] -> w219
      frame False {
        n119 = Wait Until Next ms Multiple(millisecond multiple=u32 500) -> ()  [unwired: 1 out]
      }
      frame True {
      }
    }
    n120 = call "IMAQ Rotate"("Angle (degrees)"=sgl 180.0, "Image Src"=w219) -> ("Image Dst Out"=→"Camera Image 2":T1)  [unwired: 8 in, 1 out]
  }
  n121 = while {
    tunnel: w52 -> [w245]
    tunnel: w30 -> [w243]
    tunnel: [w241] -> _
    tunnel: u32 1000 ("milliseconds to wait") -> [w240]
    tunnel: w21 -> [w234]
    i -> [w241]
    stop <- FALSE stop-if-true
    n122 = local read "Rec Mode"() -> (w236:enum32{"Stop", "Record", "Playback"})
    n123 = Wait on Notification(notifier=w243, timeout in ms (-1)=w240) -> (notification=w242:string, timed out?=w238:bool)  [unwired: 2 in, 2 out]
    n124 = Equal?(x=w236, y=u16 2 ("Rec Mode")) -> (x = y?=w237:bool)
    n125 = Compound Arithmetic op=OR(invert w238, w237) -> (w239:bool)
    n126 = case shown="True" w239 {
      tunnel: w245 -> [_ w248]
      tunnel: w242 -> [_ w247]
      tunnel: w234 -> [_ w246]
      frame False {
      }
      frame True {
        n127 = call <vilib>:"Bind Controls to SmartDashboard.vi"("RPC ref"=w246, "Bound Control Refs"=w248, "Server IP Address"=w247) -> ()  [unwired: 9 in]
      }
    }
  }
  n128 = while {
    tunnel: w71 -> [w258]
    tunnel: w70 -> [_]
    tunnel: [w259] -> _
    i -> [w259]
    stop <- FALSE stop-if-true
    # "Optionally read the DB image,\nlog, or retrieve images from a\nlogged match"
    n129 = local read "Rec Mode"() -> (w254:enum32{"Stop", "Record", "Playback"})
    n130 = local read "Robot IP"() -> (w253:string)
    n131 = call <vilib>:"WPI_CameraRead MJPG for Dashboard.vi"("Camera Settings"="Camera Settings", "Rec Mode"=w254, "Robot IP"=w253, "Camera Name"="Camera Name", "Refnum in"=w258) -> ("Active"=w256:bool, "Refnum out"=w257:T1, "FPS"=w255:dbl, "Bandwidth (Mbps)"=w252:dbl)  [unwired: 3 in]
    n132 = case shown="True" w256 {
      tunnel: w257 -> [w261 w280]
      tunnel: w252 -> [_ w277]
      tunnel: w255 -> [_ w278]
      tunnel: [w261 w273] -> w249
      frame False {
        w263 = u32 1985280 ("Color Box")
        # "Sleep for 500ms"
        n133 = Bundle("Color Box"=w263, "Color Box"=w263) -> (w264:cluster{"Color Box":u32, "Color Box":u32})  [unwired: 1 out]
        n134 = Build Array(w264) -> (w262:cluster{"Color Box":u32, "Color Box":u32}[])
        n135 = property on="Mbps LED" class="Bool (strict)"("Colors [4]"=w262) -> ()  [unwired: 2 in, 2 out]
        n136 = Wait Until Next ms Multiple(millisecond multiple=u32 500) -> ()  [unwired: 1 out]
      }
      frame True {
        # "Here is where you would annotate,\npossibly process, and display the image"
        # "Update Mbps LED"
        n137 = case shown="Default" w277 {
          tunnel: [u32 6618880 ("Color Box") u32 16776722 ("Color Box") u32 16716800 ("Color Box")] -> w281
          frame Default {
          }
          frame 4, 5 {
          }
          frame 6.. {
          }
        }
        n138 = call "IMAQ Clear Overlay"("Image"=w280) -> ("error out"=w283:errorcluster, "Image Out"=w274:T1)  [unwired: 2 in, 7 out]
        n139 = Bundle(FALSE, "Bandwidth (Mbps)"=w277, "FPS"=w278) -> (→"Camera Info":cluster{bool, "Bandwidth (Mbps)":dbl, "FPS":dbl})  [unwired: 1 in]
        n140 = Bundle("Color Box"=w281, "Color Box"=w281) -> (w282:cluster{"Color Box":u32, "Color Box":u32})  [unwired: 1 out]
        n141 = Unbundle By Name(w283) -> ("status"=w284:bool)
        n142 = Build Array(w282) -> (w279:cluster{"Color Box":u32, "Color Box":u32}[])
        n143 = property on="Image Message" class="Str"("Visible"=w284) -> ()  [unwired: 2 in, 2 out]
        n144 = property on="Mbps LED" class="Bool (strict)"("Colors [4]"=w279) -> ()  [unwired: 2 in, 2 out]
        n145 = call-poly <vilib>:"NT Read Value.vi"("Name"="Vision Data") -> ("String"=w271:string)  [unwired: 9 in, 1 out]
        n146 = Unflatten From String(type="output cluster", binary string=w271) -> (value=w269:T2)  [unwired: 3 in, 2 out]
        n147 = Unbundle By Name(w269) -> ("Results"=w268:T8, "Edges"=w267:cluster{"X":sgl, "Y":sgl}[])  [unwired: 1 out]
        n148 = call "Label Targets2.vi"("Edges"=w267, "Annotate"=TRUE, "Results"=w268, "Image in"=w274) -> ("Image out"=w273:T1)  [unwired: 7 in]
      }
    }
    "Camera Image" <- w249
  }
  n149 = vi-ref "Playback Controls.vi"() -> (w61:refnum<vi>)
  n150 = property class="Pnl"(reference=w63) -> ("Panes[]"=w64:refnum<vi>[])  [unwired: 1 in, 2 out]
  n151 = Index Array(array=w64) -> (element=w62:refnum<vi>)  [unwired: 1 in]
  n152 = control-ref of="Test Tree"() -> (w65:refnum<vi>)
  n153 = while {
    tunnel: [w297] -> _
    tunnel: w65 -> [w296]
    tunnel: w61 -> [w295]
    tunnel: w60 -> [w294]
    tunnel: w59 -> [_]
    tunnel: w55 -> [w293]
    tunnel: w21 -> [w292]
    tunnel: w19 -> [w291]
    shift-right: [w290] -> _
    shift-left: _ -> [w289]
    tunnel: w13 -> [w288]
    i -> [w297]
    stop <- FALSE stop-if-true
    n154 = event shown="[0] Timeout" {
      selector: w294 -> [_ _ _ _ _ _ _ _ _ _ _ _ _ _ _ _ _ _ _ _ _]
      dyn-events: [_ _ _ _ _ _ _ _ _ _ _ _ _ _ _ _ w553 _ _ _ _] -> _
      timeout: u32 60 ("milliseconds to wait") -> [_ _ _ _ _ _ _ _ _ _ _ _ _ _ _ _ _ _ _ _ _]
      tunnel: w296 -> [w309 _ _ _ _ _ _ _ _ _ _ _ _ _ _ _ _ _ _ _ _]
      tunnel: "Test Tree" -> [_ _ _ _ _ _ _ _ _ _ _ w520 w528 w530 w534 w542 _ _ _ _ _]
      tunnel: w295 -> [_ _ _ _ _ _ _ _ _ _ _ _ _ _ _ _ w555 _ w573 _ _]
      tunnel: w293 -> [_ _ _ _ _ _ _ _ _ _ _ _ _ _ _ _ w551 _ _ _ _]
      tunnel: w292 -> [_ _ _ _ _ _ _ _ _ _ _ _ _ _ _ _ w547 _ _ _ _]
      tunnel: w291 -> [w304 _ _ _ _ _ w471 _ _ _ _ _ _ _ _ _ _ _ _ _ _]
      tunnel: [w303 w348 w450 w455 w464 w468 w469 w478 w488 w495 w507 w519 w526 w529 w533 w541 w546 w568 w570 w574 w585] -> w290
      tunnel: w289 -> [w303 w348 w450 w455 w464 w468 w469 _ _ w495 w507 w519 w526 w529 w533 w541 w546 w568 w570 w574 w585]
      tunnel: w288 -> [w301 _ _ _ _ _ _ _ _ _ _ _ _ _ _ _ _ _ _ _ _]
      event Timeout {
        n155 = event-data() -> ()  [unwired: 1 in, 1 out]
        n156 = local read "Mode"() -> (w306:T7)
        n157 = case shown="\"Custom\", Default" "Dashboard Tab" {
          tunnel: w309 -> [_ _ w325 _ _]
          tunnel: "/TestMode/Automatic/" ("Name Pattern") -> [_ _ w324 _ _]
          tunnel: T24 [{"Operation"=enum."Clear", "Color Box"=14013909}, {"Operation"=enum."Clear", "Color Box"=14013909}, {"Operation"=enum."Clear", "Color Box"=14013909}, {"Operation"=enum."Clear", "Color Box"=14013909}, {"Operation"=enum."Update", "Color Box"=14013909}, {"Operation"=enum."Update", "Color Box"=16777215}, {"Operation"=enum."Clear", "Color Box"=14013909}, {"Operation"=enum."Clear", "Color Box"=14013909}, {"Operation"=enum."Clear", "Color Box"=14013909}] -> [_ _ w317 _ w341]
          tunnel: w306 -> [_ _ w316 _ w340]
          tunnel: u32[] [15790320, 15790320, 15790320, 15790320, 16777215, 16777215, 15790320, 15790320, 15790320] -> [_ _ _ _ w346]
          tunnel: w304 -> [_ _ _ _ w334]
          tunnel: w301 -> [_ w311 _ _ _]
          frame "Custom", Default {
          }
          frame "Basic" {
            n158 = call <vilib>:"WPI_DashboardUpdateNames.vi"("Controls on Tab"=w311) -> ()  [unwired: 11 in]
          }
          frame "Test" {
            w323 = -2 ("Active Item:Row Number")
            n159 = Index Array(array=w317, index=w316) -> (element=w318:T27)
            n160 = Unbundle(w318) -> ("Operation"=w319:enum16{"Update", "Clear"}, "Color Box"=w320:u32)
            n161 = call <vilib>:"NT Read String.vi"("Name"="/TestMode/TestName") -> ("String"=w314:string)  [unwired: 9 in, 1 out]
            n162 = call <vilib>:"NT Read and Format Entries as Tree.vi"("Operation"=w319, "Name Pattern"=w324, "Tree Refnum"=w325) -> ()  [unwired: 7 in, 2 out]
            n163 = case shown="\"\"" w314 {
              tunnel: "/TestMode/TestProgress" ("Name") -> [w327 _]
              tunnel: "/TestMode/TestProgressText" ("Name") -> [w326 _]
              frame Default {
                n164 = call <vilib>:"NT Read Number.vi"("Name"=w327) -> ("Numeric"=w328:dbl)  [unwired: 9 in, 1 out]
                n165 = call <vilib>:"NT Read String.vi"("Name"=w326) -> ("String"=w329:string)  [unwired: 9 in, 1 out]
                n166 = Bundle("Numeric"=w328, "String"=w329) -> (→"Progress":cluster{"Numeric":dbl, "String":string})  [unwired: 1 in]
              }
              frame "" {
                n167 = property on="Progress" class="Clust (strict)"("Visible"=FALSE) -> ()  [unwired: 2 in, 2 out]
                n168 = local write "Test Name"(u16 0) -> ()
              }
            }
            n169 = property on="Test Tree" class="Tree (strict)"("Active Item Row Number"=w323, "ActiveColNum"=w323, "CellBG"=w320, "Active Item Row Number"=-1 ("Active Item:Row Number"), "CellBG"=u32 5789784 ("Color Box")) -> ()  [unwired: 2 in, 2 out]
          }
          frame "Variables" {
            n170 = control-ref of="Tree"() -> (w333:refnum<vi>)
            n171 = call <vilib>:"NT Read and Format Entries as Tree.vi"("Tree Refnum"=w333) -> ()  [unwired: 9 in, 2 out]
          }
          frame "Commands" {
            w342 = u32 5789784 ("Color Box")
            w343 = T28 {"Row"=-1, "Column"=-2} ("Active Cell:Active Cell")
            w345 = T28 {"Row"=-2, "Column"=-2} ("Active Cell:Active Cell")
            n172 = Index Array(array=w346, index=w340) -> (element=w344:u32)
            n173 = Index Array(array=w341, index=w340) -> (element=w339:T27)
            n174 = Unbundle(w339) -> ("Operation"=w338:enum16{"Update", "Clear"})  [unwired: 1 out]
            n175 = local read "Command Selection"() -> (w337:i32)
            n176 = property on="Command Selection" class="MCListbox (strict)"("ActiveCell"=w345, "CellBG"=w344, "ActiveCell"=w343, "CellBG"=w342) -> ()  [unwired: 2 in, 2 out]
            n177 = call <vilib>:"WPI_DashboardUpdate RPC Info.vi"("Operation"=w338) -> ("update"=w336:bool, "commands"=w335:string[][])  [unwired: 9 in]
            n178 = property on="Command Selection" class="MCListbox (strict)"("ItemNames"=w335) -> ()  [unwired: 2 in, 2 out]
            n179 = property on="Command Params" class="Tbl (strict)"("Active Cell"=w345, "Cell BG Color"=w344, "Active Cell"=w343, "Cell BG Color"=w342) -> ()  [unwired: 2 in, 2 out]
            n180 = call <vilib>:"WPI_DashboardUpdate Command Params.vi"("Update"=w336, "NewVal"=w337, "Commands"=w335, "Param Tbl"=w334) -> ()  [unwired: 7 in, 1 out]
          }
        }
        n181 = call <vilib>:"Connextion Info.vi"() -> ("Connected"=→"NT Connection":bool)  [unwired: 10 in, 1 out]
      }
      event "Test Tree": Value Change {
        # "Show appropriate\ncontrols"
        n182 = event-data() -> ("CtlRef"=w351:refnum<vi>, "NewVal"=w349:string)  [unwired: 1 in]
        n183 = call <vilib>:"WPI_UtilitiesGetTreeIOName.vi"("NewVal"=w349, "TreeControl in"=w351) -> ("I/O Name"=w352:string)  [unwired: 9 in]
        n184 = case shown="\"Servo\"" w352 {
          selector: w352 -> [_ w359 _ w381 w390 _]
          tunnel: w349 -> [_ _ w378 w380 _ w397]
          tunnel: cluster{string[]}[] [{["640x480", "320x240", "160x120"]}, {["Auto", "Fixed indoor", "Fixed outdoor 1", "Fixed outdoor 2", "Fixed fluorescent 1", "Fixed fluorescent 2", "Hold current"]}, {["Auto", "Flicker-free 50 Hz", "Flicker-free 60 Hz", "Hold current"]}, {["None", "Prioritize frame rate", "Prioritize image quality"]}, {["Monochrome", "Color"]}] -> [_ _ _ _ _ w396]
          frame Default {
            w354 = FALSE ("Visible")
            w353 = FALSE ("Visible")
            n185 = property on="Motor" class="Clust (strict)"("Visible"=w353) -> ()  [unwired: 2 in, 2 out]
            n186 = property on="Test Ring" class="Ring (strict)"("Visible"=w353) -> ()  [unwired: 2 in, 2 out]
            n187 = property on="Rev/Fwd" class="Clust (strict)"("Visible"=w354) -> ()  [unwired: 2 in, 2 out]
            n188 = property on="On/Off" class="Bool (strict)"("Visible"=w354) -> ()  [unwired: 2 in, 2 out]
            n189 = property on="Test Slider" class="Slide (strict)"("Visible"=w354) -> ()  [unwired: 2 in, 2 out]
          }
          frame "Analog Out", "Motor", "PWM" {
            w360 = FALSE ("Visible")
            n190 = case shown="\"Analog Out\"" w359 {
              tunnel: [1.0 ("Value") -1.0 ("Value") 0.0 ("Value")] -> w358
              tunnel: [255.0 ("Value") 1.0 ("Value") 5.0 ("Value")] -> w357
              tunnel: [128.0 ("Value") 0.0 ("Value") 0.0 ("Value")] -> w356
              tunnel: [64.0 ("Value") 0.5 ("Value") 1.0 ("Value")] -> w355
              frame "PWM" {
              }
              frame "Motor", Default {
              }
              frame "Analog Out" {
              }
            }
            n191 = property on="Motor" class="Clust (strict)"("Visible"=TRUE) -> ()  [unwired: 2 in, 2 out]
            n192 = property on="Value" class="Slide (strict)"("Value"=w356, "Scale.Minimum"=w358, "Scale.Maximum"=w357, "Scale.Increment"=w355) -> ()  [unwired: 2 in, 2 out]
            n193 = property on="On/Off" class="Bool (strict)"("Visible"=w360) -> ()  [unwired: 2 in, 2 out]
            n194 = property on="Test Slider" class="Slide (strict)"("Visible"=w360) -> ()  [unwired: 2 in, 2 out]
            n195 = property on="Test Ring" class="Ring (strict)"("Visible"=w360) -> ()  [unwired: 2 in, 2 out]
            n196 = property on="Rev/Fwd" class="Clust (strict)"("Visible"=w360) -> ()  [unwired: 2 in, 2 out]
          }
          frame "Servo" {
            w376 = FALSE ("Visible")
            n197 = call <vilib>:"NT Read Number.vi"("Name"=w378) -> ("Numeric"=w377:dbl)  [unwired: 9 in, 1 out]
            n198 = property on="Test Slider" class="Slide (strict)"("Visible"=TRUE, "Scale.Maximum"=170.0 ("Scale.Range:Maximum")) -> ()  [unwired: 2 in, 2 out]
            n199 = local write "Test Slider"(w377) -> ()
            n200 = property on="Motor" class="Clust (strict)"("Visible"=w376) -> ()  [unwired: 2 in, 2 out]
            n201 = property on="Rev/Fwd" class="Clust (strict)"("Visible"=w376) -> ()  [unwired: 2 in, 2 out]
            n202 = property on="On/Off" class="Bool (strict)"("Visible"=w376) -> ()  [unwired: 2 in, 2 out]
            n203 = property on="Test Ring" class="Ring (strict)"("Visible"=w376) -> ()  [unwired: 2 in, 2 out]
          }
          frame "Relay", "Solenoid" {
            w379 = FALSE ("Visible")
            n204 = property on="Motor" class="Clust (strict)"("Visible"=w379) -> ()  [unwired: 2 in, 2 out]
            n205 = property on="Test Slider" class="Slide (strict)"("Visible"=w379) -> ()  [unwired: 2 in, 2 out]
            n206 = Search and Replace String(input string=w380, search string="/Value  **", replace string="/Direction") -> (result string=w386:string)  [unwired: 5 in, 3 out]
            n207 = property on="Test Ring" class="Ring (strict)"("Visible"=w379) -> ()  [unwired: 2 in, 2 out]
            n208 = call <vilib>:"NT Read String.vi"("Name"=w386) -> ("String"=w384:string)  [unwired: 9 in, 1 out]
            n209 = Equal?(x="Both directions", y=w384) -> (x = y?=w382:bool)
            n210 = Not(x=w382) -> (.not. x?=w383:bool)
            n211 = property on="Rev/Fwd" class="Clust (strict)"("Visible"=w382) -> ()  [unwired: 2 in, 2 out]
            n212 = property on="On/Off" class="Bool (strict)"("Visible"=w383, "Caption.Text"=w381) -> ()  [unwired: 2 in, 2 out]
          }
          frame "Compressor", "Digital Out" {
            w389 = FALSE ("Visible")
            # "Get direction and finish"
            n213 = property on="Motor" class="Clust (strict)"("Visible"=w389) -> ()  [unwired: 2 in, 2 out]
            n214 = property on="Test Slider" class="Slide (strict)"("Visible"=w389) -> ()  [unwired: 2 in, 2 out]
            n215 = property on="Test Ring" class="Ring (strict)"("Visible"=w389) -> ()  [unwired: 2 in, 2 out]
            n216 = property on="On/Off" class="Bool (strict)"("Visible"=TRUE, "Caption.Text"=w390) -> ()  [unwired: 2 in, 2 out]
            n217 = property on="Rev/Fwd" class="Clust (strict)"("Visible"=FALSE) -> ()  [unwired: 2 in, 2 out]
          }
          frame "Camera" {
            n218 = call <vilib>:"Get Last Path Segment.vi"("String in"=w397) -> ("String out"=w398:string)  [unwired: 10 in]
            n219 = property on="On/Off" class="Bool (strict)"("Visible"=FALSE) -> ()  [unwired: 2 in, 2 out]
            n220 = property on="Motor" class="Clust (strict)"("Visible"=FALSE) -> ()  [unwired: 2 in, 2 out]
            n221 = property on="Rev/Fwd" class="Clust (strict)"("Visible"=FALSE) -> ()  [unwired: 2 in, 2 out]
            n222 = case shown="\"Brightness  **\", \"Color Level  **\", \"Compression  **\", \"FPS  **\", \"Sharpness  **\"" w398 {
              tunnel: w397 -> [w404 w413 w422 w431 w440 _ w446]
              tunnel: w396 -> [w402 w410 w419 w428 w437 _ _]
              frame "Size  **" {
                n223 = Index Array(array=w402) -> (element=w401:cluster{string[]})  [unwired: 1 in]
                n224 = call <vilib>:"NT Read String.vi"("Name"=w404) -> ("String"=w403:string)  [unwired: 9 in, 1 out]
                n225 = Unbundle(w401) -> (w399:string[])
                n226 = Match First String(2:w399, 3:w403) -> (0:w400:i32)  [unwired: 1 out]
                n227 = property on="Test Ring" class="Ring (strict)"("Value"=w400, "Strings []"=w399) -> ()  [unwired: 2 in, 2 out]
                n228 = property on="Test Ring" class="Ring (strict)"("Visible"=TRUE) -> ()  [unwired: 2 in, 2 out]
                n229 = property on="Test Slider" class="Slide (strict)"("Visible"=FALSE) -> ()  [unwired: 2 in, 2 out]
              }
              frame "White Balance  **" {
                n230 = Index Array(array=w410, index=1) -> (element=w411:cluster{string[]})
                n231 = call <vilib>:"NT Read String.vi"("Name"=w413) -> ("String"=w412:string)  [unwired: 9 in, 1 out]
                n232 = Unbundle(w411) -> (w408:string[])
                n233 = Match First String(2:w408, 3:w412) -> (0:w407:i32)  [unwired: 1 out]
                n234 = property on="Test Ring" class="Ring (strict)"("Value"=w407, "Strings []"=w408) -> ()  [unwired: 2 in, 2 out]
                n235 = property on="Test Ring" class="Ring (strict)"("Visible"=TRUE) -> ()  [unwired: 2 in, 2 out]
                n236 = property on="Test Slider" class="Slide (strict)"("Visible"=FALSE) -> ()  [unwired: 2 in, 2 out]
              }
              frame "Exposure  **" {
                n237 = Index Array(array=w419, index=2) -> (element=w420:cluster{string[]})
                n238 = call <vilib>:"NT Read String.vi"("Name"=w422) -> ("String"=w421:string)  [unwired: 9 in, 1 out]
                n239 = Unbundle(w420) -> (w416:string[])
                n240 = Match First String(2:w416, 3:w421) -> (0:w417:i32)  [unwired: 1 out]
                n241 = property on="Test Ring" class="Ring (strict)"("Value"=w417, "Strings []"=w416) -> ()  [unwired: 2 in, 2 out]
                n242 = property on="Test Ring" class="Ring (strict)"("Visible"=TRUE) -> ()  [unwired: 2 in, 2 out]
                n243 = property on="Test Slider" class="Slide (strict)"("Visible"=FALSE) -> ()  [unwired: 2 in, 2 out]
              }
              frame "Exposure Priority  **" {
                n244 = Index Array(array=w428, index=3) -> (element=w429:cluster{string[]})
                n245 = call <vilib>:"NT Read String.vi"("Name"=w431) -> ("String"=w430:string)  [unwired: 9 in, 1 out]
                n246 = Unbundle(w429) -> (w425:string[])
                n247 = Match First String(2:w425, 3:w430) -> (0:w426:i32)  [unwired: 1 out]
                n248 = property on="Test Ring" class="Ring (strict)"("Value"=w426, "Strings []"=w425) -> ()  [unwired: 2 in, 2 out]
                n249 = property on="Test Ring" class="Ring (strict)"("Visible"=TRUE) -> ()  [unwired: 2 in, 2 out]
                n250 = property on="Test Slider" class="Slide (strict)"("Visible"=FALSE) -> ()  [unwired: 2 in, 2 out]
              }
              frame "Color Enable  **" {
                n251 = Index Array(array=w437, index=4) -> (element=w438:cluster{string[]})
                n252 = call <vilib>:"NT Read String.vi"("Name"=w440) -> ("String"=w439:string)  [unwired: 9 in, 1 out]
                n253 = Unbundle(w438) -> (w434:string[])
                n254 = Match First String(2:w434, 3:w439) -> (0:w435:i32)  [unwired: 1 out]
                n255 = property on="Test Ring" class="Ring (strict)"("Value"=w435, "Strings []"=w434) -> ()  [unwired: 2 in, 2 out]
                n256 = property on="Test Ring" class="Ring (strict)"("Visible"=TRUE) -> ()  [unwired: 2 in, 2 out]
                n257 = property on="Test Slider" class="Slide (strict)"("Visible"=FALSE) -> ()  [unwired: 2 in, 2 out]
              }
              frame Default {
                n258 = property on="Test Ring" class="Ring (strict)"("Visible"=FALSE) -> ()  [unwired: 2 in, 2 out]
                n259 = property on="Test Slider" class="Slide (strict)"("Visible"=FALSE) -> ()  [unwired: 2 in, 2 out]
              }
              frame "Brightness  **", "Color Level  **", "Compression  **", "FPS  **", "Sharpness  **" {
                n260 = call <vilib>:"NT Read Number.vi"("Name"=w446) -> ("Numeric"=w445:dbl)  [unwired: 9 in, 1 out]
                n261 = local write "Test Slider"(w445) -> ()
                n262 = property on="Test Slider" class="Slide (strict)"("Visible"=TRUE, "Scale.Maximum"=100.0 ("Scale.Range:Maximum")) -> ()  [unwired: 2 in, 2 out]
                n263 = property on="Test Ring" class="Ring (strict)"("Visible"=FALSE) -> ()  [unwired: 2 in, 2 out]
              }
            }
          }
        }
        n264 = property on="Progress" class="Clust (strict)"("Visible"=FALSE) -> ()  [unwired: 2 in, 2 out]
      }
      event "Test Name": Mouse Enter {
        # "Populate the ring with the list of tests"
        n265 = event-data() -> ()  [unwired: 1 in, 1 out]
        n266 = call <vilib>:"NT Read String Array.vi"("Name"="/TestMode/TestList") -> ("String Array"=w454:string[])  [unwired: 9 in, 1 out]
        n267 = Build Array (concatenate)("Select the test to run...", w454) -> (w453:string[])
        n268 = property on="Test Name" class="Ring (strict)"("Strings []"=w453) -> ()  [unwired: 2 in, 2 out]
      }
      event "Test Name": Value Change {
        w456 = FALSE ("Visible")
        # "Tell the robot the test name to run"
        n269 = event-data() -> ("NewVal"=w460:u16)  [unwired: 1 in]
        n270 = property on="Test Name" class="Ring (strict)"() -> ("Strings []"=w461:string[])  [unwired: 2 in, 2 out]
        n271 = local write "Progress"(T9 {"Test Progress"=0, "Test Progress Text"=""} ("Progress")) -> ()
        n272 = Index Array(array=w461, index=w460) -> (element=w459:string)
        n273 = call <vilib>:"NT Write String.vi"("String"=w459, "Name"="/TestMode/TestName") -> ()  [unwired: 9 in, 1 out]
        n274 = property on="Progress" class="Clust (strict)"("Visible"=TRUE) -> ()  [unwired: 2 in, 2 out]
        n275 = property on="Motor" class="Clust (strict)"("Visible"=w456) -> ()  [unwired: 2 in, 2 out]
        n276 = property on="Test Slider" class="Slide (strict)"("Visible"=w456) -> ()  [unwired: 2 in, 2 out]
        n277 = property on="On/Off" class="Bool (strict)"("Visible"=w456) -> ()  [unwired: 2 in, 2 out]
        n278 = property on="Rev/Fwd" class="Clust (strict)"("Visible"=w456) -> ()  [unwired: 2 in, 2 out]
        n279 = property on="Test Ring" class="Ring (strict)"("Visible"=w456) -> ()  [unwired: 2 in, 2 out]
      }
      event "Select Auto": Mouse Enter {
        # "Populate the combo box with the list of autonomous options"
        n280 = event-data() -> ()  [unwired: 1 in, 1 out]
        n281 = call <vilib>:"NT Read String Array.vi"("Name"="Auto List") -> ("String Array"=w463:string[])  [unwired: 9 in, 1 out]
        n282 = property on="Select Auto" class="CmbBox"("Strings[]"=w463) -> ()  [unwired: 2 in, 2 out]
      }
      event "Select Auto": Value Change {
        # "User modified the Auto Selection. Write to NT variable so robot knows."
        n283 = event-data() -> ("NewVal"=w466:string)  [unwired: 1 in]
        n284 = call <vilib>:"NT Write String.vi"("String"=w466, "Name"="Auto Selector") -> ()  [unwired: 9 in, 1 out]
      }
      event "Command Selection": Value Change {
        # "Get the params and show in table"
        n285 = event-data() -> ("NewVal"=w472:i32)  [unwired: 1 in]
        n286 = property on="Command Selection" class="MCListbox (strict)"() -> ("ItemNames"=w470:string[][])  [unwired: 2 in, 2 out]
        n287 = call <vilib>:"WPI_DashboardUpdate Command Params.vi"("NewVal"=w472, "Commands"=w470, "Param Tbl"=w471) -> ()  [unwired: 8 in, 1 out]
      }
      event "Execute Command": Value Change {
        # "Started one, Unique ID holds\nresponse"
        n288 = event-data() -> ()  [unwired: 1 in, 1 out]
        n289 = property on="Command Selection" class="MCListbox (strict)"() -> ("ItemNames"=w483:string[][])  [unwired: 2 in, 2 out]
        n290 = Index Array(array=w483, index (row)="Command Selection", index (col)=0) -> (element=w481:string)
        n291 = call <vilib>:"Invoke Commands.vi"("Command Params"="Command Params", "Function Name"=w481) -> ("Params"=w477:u8, "Started"=w476:bool)  [unwired: 7 in, 1 out]
        n292 = Array Subset(array="Command Params", length (row)=w477) -> (w478:string[][])  [unwired: 3 in]
        n293 = Select(t="Executing" ("Cmd Status"), s=w476, f="" ("Cmd Status")) -> (s? t:f=→"Cmd Status":string)
      }
      event "Command Selection": Double Click {
        n294 = event-data() -> ("Row"=w491:i32)  [unwired: 1 in]
        n295 = property on="Command Selection" class="MCListbox (strict)"() -> ("ItemNames"=w494:string[][])  [unwired: 2 in, 2 out]
        n296 = local read "Command Params"() -> (w490:string[][])
        n297 = Index Array(array=w494, index (row)=w491, index (col)=0) -> (element=w492:string)
        n298 = call <vilib>:"Invoke Commands.vi"("Command Params"=w490, "Function Name"=w492) -> ("Params"=w489:u8, "Started"=w484:bool)  [unwired: 7 in, 1 out]
        n299 = Array Subset(array=w490, length (row)=w489) -> (w488:string[][])  [unwired: 3 in]
        n300 = Select(t="Executing" ("Cmd Status"), s=w484, f="" ("Cmd Status")) -> (s? t:f=w485:string)
        n301 = local write "Cmd Status"(w485) -> ()
      }
      event "CheckList": Double Click {
        # "Shift clears all"
        # "Update symbols on the listbox"
        n302 = event-data() -> ("PlatMods.Shift"=w496:bool, "Row"=w498:i32)  [unwired: 1 in]
        n303 = case shown="True" w496 {
          tunnel: w498 -> [w502 _]
          tunnel: 1 -> [w501 _]
          frame False {
            n304 = property on="CheckList" class="LstBox (strict)"() -> ("Item Symbols"=w500:i32[])  [unwired: 2 in, 2 out]
            n305 = Replace Array Subset(array=w500, new element=w501, index=w502) -> (w499:i32[])
            n306 = property on="CheckList" class="LstBox (strict)"("Item Symbols"=w499) -> ()  [unwired: 2 in, 2 out]
          }
          frame True {
            w503 = 0 ("Top Row")
            n307 = property on="CheckList" class="LstBox (strict)"() -> ("Number of Rows"=w505:u32)  [unwired: 2 in, 2 out]
            n308 = Initialize Array(0, w505) -> (w504:i32[])
            n309 = property on="CheckList" class="LstBox (strict)"("Top Row"=w503, "Value"=w503, "Item Symbols"=w504) -> ()  [unwired: 2 in, 2 out]
          }
        }
      }
      event "CheckList": Key Down {
        # "Update symbols on the listbox\nLeft and right keys check and uncheck"
        n310 = event-data() -> ("VKey"=w509:T25)  [unwired: 1 in]
        n311 = case shown="\"Left\", \"Right\"" w509 {
          selector: w509 -> [w514 _]
          tunnel: eventvkey."Left" ("VKey") -> [w512 _]
          frame "Left", "Right" {
            n312 = Equal?(x=w512, y=w514) -> (x = y?=w513:bool)
            n313 = Select(t=0, s=w513, f=1) -> (s? t:f=w515:i32)
            n314 = property on="CheckList" class="LstBox (strict)"() -> ("Item Symbols"=w518:i32[])  [unwired: 2 in, 2 out]
            n315 = Replace Array Subset(array=w518, new element=w515, index="CheckList") -> (w517:i32[])
            n316 = property on="CheckList" class="LstBox (strict)"("Item Symbols"=w517) -> ()  [unwired: 2 in, 2 out]
          }
          frame Default {
          }
        }
      }
      event "Motor.Enable": Value Change {
        # "When the test mode otor enable helper is set, update that\ntree row item's value"
        n317 = event-data() -> ("NewVal"=w524:bool)  [unwired: 1 in]
        n318 = Unbundle("Motor") -> ("Value"=w523:dbl)  [unwired: 1 out]
        n319 = Select(t=w523, s=w524, f=0.0) -> (s? t:f=w521:dbl)
        n320 = call <vilib>:"NT Write Number.vi"("Numeric"=w521, "Name"=w520) -> ()  [unwired: 9 in, 1 out]
      }
      event "Test Slider": Value Change {
        # "When the test mode slider helper is set, update that\ntree row item's value"
        n321 = event-data() -> ("NewVal"=w527:dbl)  [unwired: 1 in]
        n322 = call <vilib>:"NT Write Number.vi"("Numeric"=w527, "Name"=w528) -> ()  [unwired: 9 in, 1 out]
      }
      event "On/Off": Value Change {
        # "When the test mode on/off helper value is set, update that\ntree row item's value"
        n323 = event-data() -> ("NewVal"=w532:bool)  [unwired: 1 in]
        n324 = Boolean To (0,1)(Boolean=w532) -> (0, 1=w531:i16)
        n325 = call <vilib>:"NT Write Number.vi"("Numeric"=w531, "Name"=w530) -> ()  [unwired: 9 in, 1 out]
      }
      event "Rev/Fwd": Value Change {
        # "When the test mode helper value for relays is set, update that\ntree row item's value"
        n326 = event-data() -> ("NewVal.Forward"=w540:bool, "NewVal.Reverse"=w539:bool)  [unwired: 1 in]
        n327 = Boolean To (0,1)(Boolean=w540) -> (0, 1=w536:i16)
        n328 = Boolean To (0,1)(Boolean=w539) -> (0, 1=w538:i16)
        n329 = Negate(x=w538) -> (-x=w537:i16)
        n330 = Add(x=w536, y=w537) -> (x+y=w535:i16)
        n331 = call <vilib>:"NT Write Number.vi"("Numeric"=w535, "Name"=w534) -> ()  [unwired: 9 in, 1 out]
      }
      event "Test Ring": Value Change {
        # "When a test mode helper value is selected from the ring,\nset the tree item's variable to the string value"
        n332 = event-data() -> ("NewVal"=w544:u16)  [unwired: 1 in]
        n333 = property on="Test Ring" class="Ring (strict)"() -> ("Strings []"=w545:string[])  [unwired: 2 in, 2 out]
        n334 = Index Array(array=w545, index=w544) -> (element=w543:string)
        n335 = call <vilib>:"NT Write String.vi"("String"=w543, "Name"=w542) -> ()  [unwired: 9 in, 1 out]
      }
      event "Rec Mode": Value Change {
        # "Update globals for recording mode and path to read log from.\nClear when logging and let NetworkTables set path for vision to\nuse."
        n336 = event-data() -> ("NewVal"=w556:enum32{"Stop", "Record", "Playback"})  [unwired: 1 in]
        n337 = global write "WPI_DashboardLogging Global.vi" "Logging Filename"(path "") -> ()
        n338 = global write "WPI_DashboardLogging Global.vi" "Recording"(w556) -> ()
        n339 = case shown="\"Playback\"" w556 {
          tunnel: w555 -> [_ w558 w567]
          tunnel: [_ _ w566] -> w553
          tunnel: [_ _ w565] -> _
          tunnel: w551 -> [_ _ w563]
          tunnel: cluster{i32, i32} {-250, 170} -> [_ _ w562]
          tunnel: [_ _ T26 {"Image Size"=TRUE, "Image Type"=TRUE, "Pixel Value"=TRUE, "ROI Information"=TRUE, "Zoom Factor"=FALSE} ("Image Information Shown:All Elements")] -> w549
          tunnel: [_ _ TRUE ("Zoom Factor")] -> w548
          tunnel: w547 -> [_ _ w559]
          frame Default {
          }
          frame "Stop", "Record" {
            # "Place Window too"
            n340 = invoke class="VI" method="FP.Close"(reference=w558) -> (reference out=w557:refnum<vi>)  [unwired: 2 in, 2 out]
            n341 = invoke class="VI" method="Abort VI"(reference=w557) -> ()  [unwired: 2 in, 3 out]
          }
          frame "Playback" {
            n342 = call "Open Playback Panel.vi"("Offset"=w562, "DB VI Ref"=w563, "Playback in"=w567) -> ("Playback out"=w564:refnum<vi>)  [unwired: 8 in]
            n343 = register-events(w564, w559) -> (reference out=w566:refnum<event-registration>, error out=w565:errorcluster)  [unwired: 2 in]
          }
        }
        n344 = property on="Camera Image" class="ImageControl"("Image Information Shown"=w549, "Image Information Visible"=w548) -> ()  [unwired: 2 in, 2 out]
        n345 = call <vilib>:"WPI_DashboardNT Log FieldName Cache.vi"("Operation"=enum16{"Lookup/Add", "Index", "Clear"}."Clear") -> ()  [unwired: 8 in, 3 out]
      }
      event Panel Close {
        w569 = enum32{"Stop", "Record", "Playback"}."Stop" ("Rec Mode")
        # "Playback window has been closed, abort"
        n346 = event-data() -> ()  [unwired: 1 in, 4 out]
        n347 = local write "Rec Mode"(w569) -> ()
        n348 = global write "WPI_DashboardLogging Global.vi" "Recording"(w569) -> ()
      }
      event Panel Close {
        # "Abort playback window and ourself"
        n349 = event-data() -> ()  [unwired: 1 in, 4 out]
        n350 = invoke class="VI" method="FP.Close"(reference=w573) -> (reference out=w572:refnum<vi>)  [unwired: 2 in, 2 out]
        n351 = invoke class="VI" method="Abort VI"(reference=w572) -> (error out=w571:errorcluster)  [unwired: 2 in, 2 out]
        n352 = invoke class="VI" method="Abort VI"(error in=w571) -> ()  [unwired: 2 in, 3 out]
      }
      event User Event {
        n353 = event-data() -> ("IDs"=w580:cluster{"RPC field ID":u16, "Unique ID":u16}, "String"=w579:string)  [unwired: 1 in]
        n354 = Bundle("IDs"=w580, "String"=w579) -> (w578:T13)  [unwired: 1 in]
        n355 = call <vilib>:"Retrieve RPC Response.vi"("RPC Response"=w578) -> ("Output"=w576:string[][])  [unwired: 10 in]
        n356 = Build Array (concatenate)(w574, w576) -> (w575:string[][])
        n357 = local write "Command Params"(w575) -> ()
        n358 = local write "Cmd Status"("" ("Cmd Status")) -> ()
      }
      event "Tree": Double Click {
        n359 = event-data() -> ("PlatMods"=w584:T29, "Tag"=w583:string)  [unwired: 1 in]
        n360 = Unbundle(w584) -> ("Shift"=w582:bool)  [unwired: 4 out]
        n361 = Not(x=w582) -> (.not. x?=w581:bool)
        n362 = call <vilib>:"NT Update Persistence.vi"("Persistence"=w581, "Name"=w583) -> ()  [unwired: 9 in, 1 out]
      }
    }
  }
  n363 = while {
    tunnel: w62 -> [w587]
    i -> [w590]
    stop <- FALSE stop-if-true
    n364 = Wait (ms)(milliseconds to wait=u32 100) -> ()  [unwired: 1 out]
    n365 = case shown="\"Playback\"" "Rec Mode" {
      tunnel: w590 -> [_ _ w605]
      tunnel: [u32 2829099 ("Base Color") u32 11141120 ("Target Color") w594] -> w586
      frame "Stop", Default {
        # "Reset the color, extra updates don't cost much"
      }
      frame "Record" {
      }
      frame "Playback" {
        # "Playback"
        n366 = Quotient & Remainder(x=w605, y=u32 50 ("milliseconds to wait")) -> (x-y*floor(x/y)=w601:u32)  [unwired: 1 out]
        n367 = Divide(x=w601, y=u32 50 ("milliseconds to wait")) -> (x/y=w598:dbl)
        n368 = Multiply(x=6.283185307179586, y=w598) -> (x*y=w603:dbl)
        n369 = Sine(x=w603) -> (sin(x)=w602:dbl)
        n370 = Absolute Value(x=w602) -> (abs(x)=w595:dbl)
        n371 = call "Interpolate RGB Color.vi"("Proportion"=w595, "Target Color"=u32 30976, "Base Color"=u32 2829099) -> ("Result Color"=w594:u32)  [unwired: 8 in]
      }
    }
    n372 = property class="Pane"(reference=w587, "PaneColor"=w586) -> ()  [unwired: 1 in, 2 out]
  }
  n373 = local write "Dashboard Tab"(Dashboard_Tabs."Cooler Stuff" ("Dashboard Tab")) -> ()
  n374 = property on="On/Off" class="Bool (strict)"("Visible"=w31) -> ()  [unwired: 2 in, 2 out]
  n375 = property on="Motor" class="Clust (strict)"("Visible"=w31) -> ()  [unwired: 2 in, 2 out]
  n376 = property on="Progress" class="Clust (strict)"("Visible"=w31) -> ()  [unwired: 2 in, 2 out]
  n377 = property on="Test Ring" class="Ring (strict)"("Visible"=w31) -> ()  [unwired: 2 in, 2 out]
  n378 = property on="Rev/Fwd" class="Clust (strict)"("Visible"=w31) -> ()  [unwired: 2 in, 2 out]
  n379 = local write "Command Selection"(u16 0 ("milliseconds to wait")) -> ()
  n380 = local write "Command Params"(string[][] [] ("Command Params")) -> ()
  n381 = global write "WPI_DashboardLogging Global.vi" "Recording"(w56) -> ()
  n382 = local write "Rec Mode"(w56) -> ()
  n383 = while {
    tunnel: u16 1741 ("timeout ms (25000)") -> [w607]
    stop <- FALSE stop-if-true
    n384 = TCP Create Listener(10:w607) -> (0:w606:errorcluster, 3:w608:refnum<k5>)  [unwired: 4 in, 1 out]
    n385 = case shown="No Error" w606 {
      selector: w606 -> [w610 _]
      tunnel: w608 -> [w611 _]
      frame No Error {
        n386 = while {
          tunnel: w611 -> [w614]
          tunnel: w610 -> [w613]
          stop <- FALSE stop-if-true
          n387 = TCP Wait On Listener(8:w613, 11:w614) -> (0:w615:errorcluster, 4:w616:refnum<k5>)  [unwired: 2 in, 3 out]
          n388 = local write "TCP"(w616) -> ()
          n389 = case shown="No Error" w615 {
            frame No Error {
            }
            frame Error {
              n390 = Wait (ms)(milliseconds to wait=u32 1000) -> ()  [unwired: 1 out]
            }
          }
        }
      }
      frame Error {
        n391 = Wait (ms)(milliseconds to wait=u32 1000) -> ()  [unwired: 1 out]
      }
    }
  }
